vi "BIAS.vi"() -> ()   [LabVIEW 2010]
uses:
  <userlib>/bias2/subvis/Imaging_State.ctl
  <vilib>/Utility/error.llb/DialogType.ctl
  <userlib>/bias2/subvis/ROI_rect.ctl
  <userlib>/BIAS2/subvis/ExposureSettings.ctl
  <vilib>/event_ctls.llb/lveventtype.ctl
  <userlib>/BIAS2/classes/CameraBase/CameraBase.lvclass
  <vilib>/addons/h5labview/H5File.lvlib
  <vilib>/addons/h5labview/H5F_mode.ctl
  <vilib>/addons/h5labview/H5GroupObject.lvlib
  <vilib>/addons/h5labview/H5Attrib.lvlib
  <vilib>/addons/h5labview/H5Base.lvlib
  <vilib>/Analysis/NI_AALPro.lvlib
  <vilib>/Utility/file.llb/Read From Spreadsheet File (DBL).vi
  <userlib>/bias2/subvis/Frame_Controls.ctl
panel:
  in  "files":T1 caption="Files"
  in  "stop":bool
  in  "fit_buttons":cluster{"selection":bool, "stored":bool} caption="Fit"
  in  "tools_zoom":T2 caption="Zoom tools"
  in  "tools_view":cluster{"sel":bool, "in":bool, "out":bool} caption="View tools"
  in  "capture":T3 caption="Capture"
  out "stop_time":dbl=11.582550000000003
  out "busy":bool caption="Busy"
  out "recent_error":bool caption="Error"
  out "remote":bool caption="Remote"
  out "attribs":variant[](array[variant])=[variant(i32 864), variant(i32 519), variant(i32 1176), variant(i32 878), variant(i64 0), variant(string "Freerun"), variant(u32 1), variant(u32 1), variant(i64 864), variant(i64 519), variant(i64 312), variant(i64 359), variant(dbl 100000.00149011612)]
  out "acquiring":bool caption="Acquiring"
  out "img_OD":T4(plugin-control)
  out "n_atoms":dbl caption="Atom number:" format="%_4e"
  out "image_raw":sgl[][](array[numeric])
  in  "tabs":T5(tab)
  in  "newinst":bool
  in  "effective_pixel":dbl caption="effective pixel size"
  in  "rotation":u16(ring) items=["Do not rotate", "Rotate 90°", "Rotate 180°", "Rotate -90°"]
  out "cam_params":cluster{"String":string, "value":variant}[](array[cluster])=[{"String"="TriggerSource", "value"=variant(string "Freerun")}, {"String"="Timeout", "value"=variant(u32 23583)}, {"String"="ShiftPixelBits", "value"=variant(bool FALSE)}, {"String"="PixelFormat", "value"=variant(string "Mono14")}] caption="Camera Parameters"
  in  "config_cam":bool
  in  "bin_y":u8=1
  in  "bin_x":u8=1
  in  "rois":T7(array[cluster])=[{"get"=FALSE, "set"=FALSE, "rect"={"left"=0, "top"=0, "right"=0, "bottom"=0}, "color"=16777224}, {"get"=FALSE, "set"=FALSE, "rect"={"left"=0, "top"=0, "right"=0, "bottom"=0}, "color"=6618880}, {"get"=FALSE, "set"=FALSE, "rect"={"left"=0, "top"=0, "right"=0, "bottom"=0}, "color"=16776960}, {"get"=FALSE, "set"=FALSE, "rect"={"left"=0, "top"=0, "right"=0, "bottom"=0}, "color"=4849919}]
  in  "camera name":string
  out "camera model":string="GX1920 (02-2410B), serial 0xF3101FDAB"
  in  "exposure":sgl=100.0 caption="exposure (ms)"
  out "location":string caption="camera location"
  out "roi_sensor":T6={"left"=0, "top"=0, "right"=1936, "bottom"=1456} caption="camera size"
  out "keep":u8
  in  "pedestal":u16=100 caption="Camera pedestal value"
  in  "comp_Isat":bool caption="compute?"
  in  "Isat":dbl=1.5
  in  "Icutoff":dbl=500.0 caption="Intensity threshold"
  in  "xsection":dbl=2.9049e-13 caption="Transition Cross-section"
  out "working dir":path
  out "current file":string
  in  "comp_list":i32(listbox) caption="Computed Frames"
  in  "raw_ctrls":T8={"col_scheme"=0, "val_min"=100.0, "val_max"=13807.0, "automax"=TRUE} {"col_scheme" items=["Grayscale", "Rainbow", "Temperature", "-", "AlpineColors", "Amherst", "Aquamarine", "ArmyColors", "AtlanticColors", "AuroraColors", "AvocadoColors", "BeachColors", "BlueGreenYellow", "BrassTones", "BrightBands", "BrownCyanTones", "CandyColors", "CherryTones", "CMYKColors", "CoffeeTones", "DarkBands", "DarkRainbow", "DarkTerrain", "DeepSeaColors", "Default", "FallColors", "FruitPunchColors", "FuchsiaTones", "GrayTones", "GrayYellowTones", "GreenBrownTerrain", "GreenPinkTones", "IslandColors", "LabVIEW", "LakeColors", "LightTemperatureMap", "LightTerrain", "MintColors", "NeonColors", "NIST", "Pastel", "PearlColors", "PigeonTones", "PlumColors", "Rainbow", "RedBlueTones", "RedGreenSplit", "RoseColors", "RustTones", "SandyTerrain", "SiennaTones", "SolarColors", "SouthwestColors", "StarryNightColors", "SunsetColors", "TemperatureMap", "ThermometerColors", "ValentineTones", "WatermelonColors"]; "val_max" format="%_4g"; "val_min" format="%_4g"}
  in  "comp_ctrls":T8={"col_scheme"=39, "val_min"=0.0, "val_max"=3.0, "automax"=FALSE} {"col_scheme" items=["Grayscale", "Rainbow", "Temperature", "-", "AlpineColors", "Amherst", "Aquamarine", "ArmyColors", "AtlanticColors", "AuroraColors", "AvocadoColors", "BeachColors", "BlueGreenYellow", "BrassTones", "BrightBands", "BrownCyanTones", "CandyColors", "CherryTones", "CMYKColors", "CoffeeTones", "DarkBands", "DarkRainbow", "DarkTerrain", "DeepSeaColors", "Default", "FallColors", "FruitPunchColors", "FuchsiaTones", "GrayTones", "GrayYellowTones", "GreenBrownTerrain", "GreenPinkTones", "IslandColors", "LabVIEW", "LakeColors", "LightTemperatureMap", "LightTerrain", "MintColors", "NeonColors", "NIST", "Pastel", "PearlColors", "PigeonTones", "PlumColors", "Rainbow", "RedBlueTones", "RedGreenSplit", "RoseColors", "RustTones", "SandyTerrain", "SiennaTones", "SolarColors", "SouthwestColors", "StarryNightColors", "SunsetColors", "TemperatureMap", "ThermometerColors", "ValentineTones", "WatermelonColors"]; "val_max" format="%_4g"; "val_min" format="%_4g"}
  in  "raw_list":i32(listbox)=-1 caption="Raw Frames"
  in  "alpha":dbl=1.0 caption="Alpha"
  in  "hold_frames":bool caption="Hold last flat/dark frames"
  in  "histograms":bool caption="Histograms"
  in  "fit_function":enum16{"Gaussian", "ThomasFermi"}(ring)
  in  "fit clip":dbl=5.0 caption="OD clip" min=1.0
  out "fit_current":bool caption="Current"
  out "fit_number":dbl caption="Fitted atom number:"
  in  "bin_size":i32=5 caption="bin size" min=1
  out "fit_params":T9(array[cluster])=[{"param"="Fit_residuals", "uncert"=0.0, "uncert 2"=0.0}, {"param"="Fit_rebin", "uncert"=0.0, "uncert 2"=0.0}, {"param"="Gaussian_X0", "uncert"=0.12302468141779599, "uncert 2"=0.0}, {"param"="Gaussian_Y0", "uncert"=0.17648801424407168, "uncert 2"=0.0}, {"param"="Gaussian_XW", "uncert"=0.11674772619735485, "uncert 2"=0.0}, {"param"="Gaussian_YW", "uncert"=0.16283739371170114, "uncert 2"=0.0}, {"param"="Gaussian_Amp", "uncert"=0.008479207725537119, "uncert 2"=0.0}, {"param"="Gaussian_Offset", "uncert"=0.003580147540181461, "uncert 2"=0.0}, {"param"="Gaussian_Nint", "uncert"=1132011.7271960815, "uncert 2"=0.0}] caption="Fit Results" {"uncert 2" format="%#_4g"; "uncert" format="%#_4g"}
  in  "auto fit":bool caption="Auto fit"
  out "data points:":u32=7656 caption="Npoints"
  out "Y-lineout":dbl[][](graph)
  out "X-lineout":dbl[][](graph)
  in  "fit_roi":T10={"get"=FALSE, "set"=FALSE, "rect"={"left"=792, "top"=473, "right"=1233, "bottom"=911}, "color"=16711680} caption="Fitting region"
  out "recent":string[](array[string]) caption="recent log messages"
  out "state":T11 caption="system state"
  in  "last error":T12={"status"=FALSE, "code"=42, "description"="", "time"=timestamp(3029490000.67111 s since 1904-01-01)} caption="most recent error:" {"time" format="%<%H:%M:%S %d/%m/%y>T"}
  out "sequencer":T13(array[cluster])
  out "comp_data":T14(array[cluster])
  out "roi_capture":T6={"left"=686, "top"=399, "right"=1281, "bottom"=1004}
  out "roi_current":T6
  out "image_data":u16[][][](array[numeric])
  out "frame":i32=-1 caption="display_frame"
  out "fit attribs":variant[](array[variant])
  out "cam_attribs":variant
  out "BLACS port":u16
  in  "calc timeout":u32=10000
  out "raw histograms":T15(array[cluster])
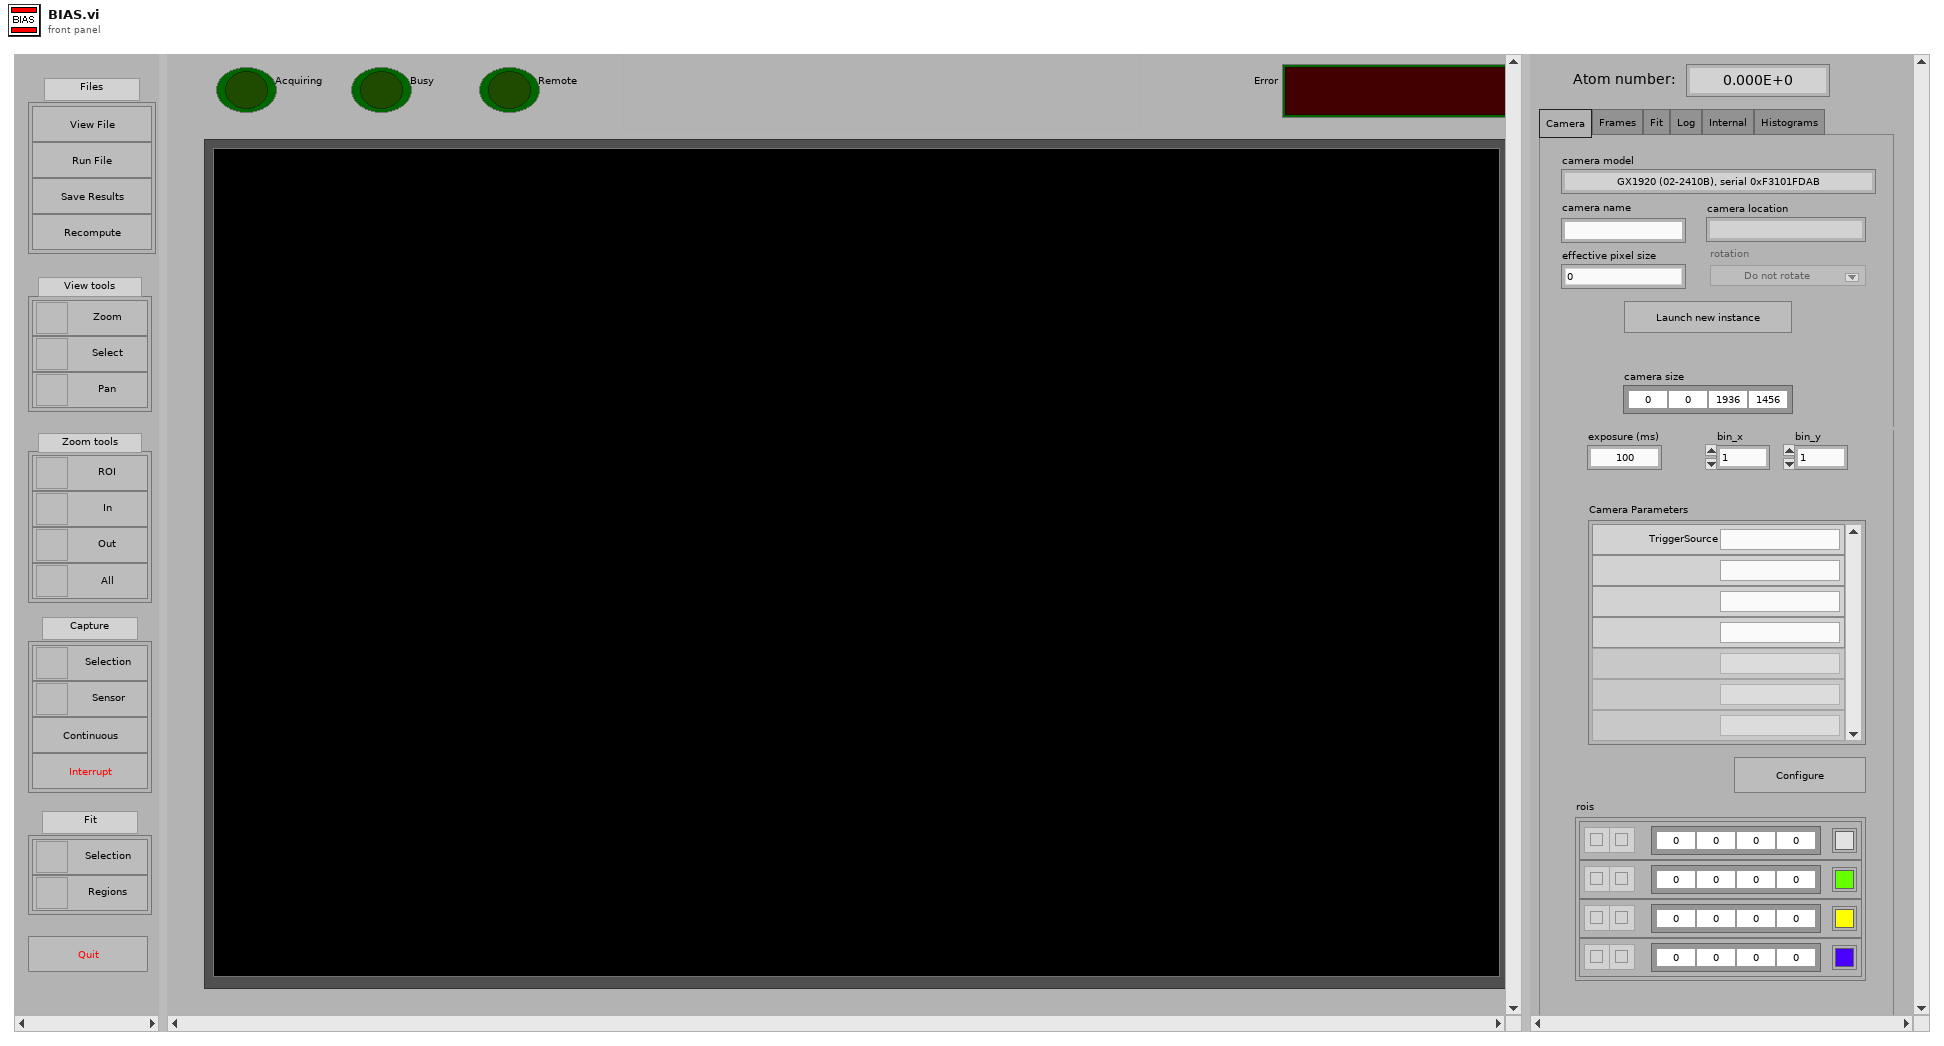
[diagram p1: front panel]
types:
  T1 = cluster{"open_file 2":bool, "open_file":bool, "save_file":bool, "open_file 3":bool}
  T2 = cluster{"sel":bool, "in":bool, "out":bool, "all":bool}
  T3 = cluster{"roi":bool, "chip":bool, "continuous":bool, "abort":bool}
  T4 = typedef "IMAQ Image.ctl" = refnum<image>
  T5 = enum32{"Camera", "Frames", "Fit", "Log", "Internal", "Histograms"}
  T6 = typedef "ROI_rect.ctl" = cluster{"left":i32, "top":i32, "right":i32, "bottom":i32}
  T7 = cluster{"get":bool, "set":bool, "rect":T6, "color":u32}[]
  T8 = typedef "Frame_Controls.ctl" = cluster{"col_scheme":u16, "val_min":sgl, "val_max":sgl, "automax":bool}
  T9 = cluster{"param":string, "uncert":dbl, "uncert 2":dbl}[]
  T10 = cluster{"get":bool, "set":bool, "rect":T6, "color":u32}
  T11 = typedef "Imaging_State.ctl" = enum16{"<NULL>", "Init", "Read File", "Save File", "Idle", "Compute", "Redraw", "Draw Overlays", "Software trigger", "Acquire", "Fit", "Clear", "Quit"}
  T12 = cluster{"status":bool, "code":i32, "description":string, "time":timestamp}
  T13 = cluster{"name":string, "shots":string[], "ids":i32[]}[]
  T14 = cluster{"sequence":string, "name":string, "data":sgl[][], "params":variant[]}[]
  T15 = cluster{"XY Graph":cluster{"X Values":dbl[], "Histogram: h(x)":i32[]}}[]
  T16 = typedef "DialogType.ctl" = u16
  T17 = typedef "zlock.ctl" = cluster{"context out":refnum<class "zmq_context.lvclass">, "endpoint":string, "timeout":u32, "name":string}
  T18 = typedef "pointer.ctl" = u64
  T19 = typedef "ExposureSettings.ctl" = cluster{"exposure":dbl, "external":bool, "roi":T6, "frames":i32, "bin_x":u8, "bin_y":u8}
  T20 = cluster{"Icutoff":dbl, "Isat":dbl, "sigma":dbl, "pixel_size":dbl}
  T21 = typedef "H5File.lvlib/H5F_mode.ctl" = enum16{"read-only", "read-write", "overwrite", "create new", "open or create"}
  T22 = enum8{"Enabled", "Disabled", "Disabled and Grayed Out"}
  T23 = typedef "Image Type" = u32
  T24 = cluster{"sensor_width":u16, "sensor_width":u16, "sensor_width":u16, "sensor_height":u16}
  T25 = cluster{"sequence":string, "name":string, "data":sgl[][], "params":variant[]}
  T26 = cluster{"X Values":dbl[], "Histogram: h(x)":i32[]}
  T27 = cluster{"Histogram Graph":cluster{"X Values":dbl[], "Histogram: h(x)":i32[]}}
  T28 = cluster{"name":string, "shots":string[], i32[]}[]
  T29 = cluster{"Name":string, "Name":string, "data":sgl[][], "params":variant[]}[]
  T30 = enum32{"Invalid", "Standard", "Closed", "Hidden", "Minimized", "Maximized"}
  T31 = typedef "lveventtype.ctl" = enum32{"Null", "Timeout", "App Instance Close", "App Instance Close?", "Autoscale Range Change", "Cell Edit", "Cell Edit?", "Cursor Grab", "Cursor Grab?", "Cursor Move", "Cursor Release", "Data Change", "Direction Change", "Display State Change", "Drag Ended", "Drag Enter", "Drag Leave", "Drag Over", "Drag Source Update", "Drag Starting", "Drag Starting?", "Drop", "Exec State Change", "Key Down", "Key Down?", "Key Repeat", "Key Repeat?", "Key Up", "Listbox Double Click", "Menu Activation?", "Menu Selection (App)", "Menu Selection? (App)", "Menu Selection (User)", "Mouse Down", "Mouse Down?", "Mouse Enter", "Mouse Leave", "Mouse Move", "Mouse Up", "NI Security User Change (App)", "Pane Size", "Panel Close", "Panel Close?", "Panel Resize", "Plot Attribute Change", "Scale Range Change", "Shortcut Menu Activation?", "Shortcut Menu Selection (App)", "Shortcut Menu Selection? (App)", "Shortcut Menu Selection (User)", "Tree Double Click", "Tree Drag", "Tree Drag?", "Tree Drop", "Tree Drop?", "Tree Item Close", "Tree Item Close?", "Tree Item Open", "Tree Item Open?", "Value Change"}
  T32 = cluster{"Global Rectangle":i32[], "Contours":cluster{"Contour Type":u32, "ROI Type":u32, "Points":i32[]}[]}
  T33 = typedef "ROI Descriptor" = cluster{"Global Rectangle":i32[], "Contours":cluster{"ID":enum32{"External", "Internal"}, "Type":u32, "Coordinates":i32[]}[]}
  T34 = cluster{"Contour Type":u32, "ROI Type":u32, "Points":i32[]}[]
  T35 = cluster{"FinalVal[0]":bool, "FinalVal[1]":bool, "FinalVal[2]":bool}
  T36 = cluster{"all rows[0]":dbl, "all rows[1]":dbl, "all rows[2]":dbl}
  T37 = cluster{"bin_x":u8, "bin_y":u8, "bin_x":u8, "bin_y":u8}
  T38 = enum16{"Standard", "Buffered", "CRLF", "Immediate"}
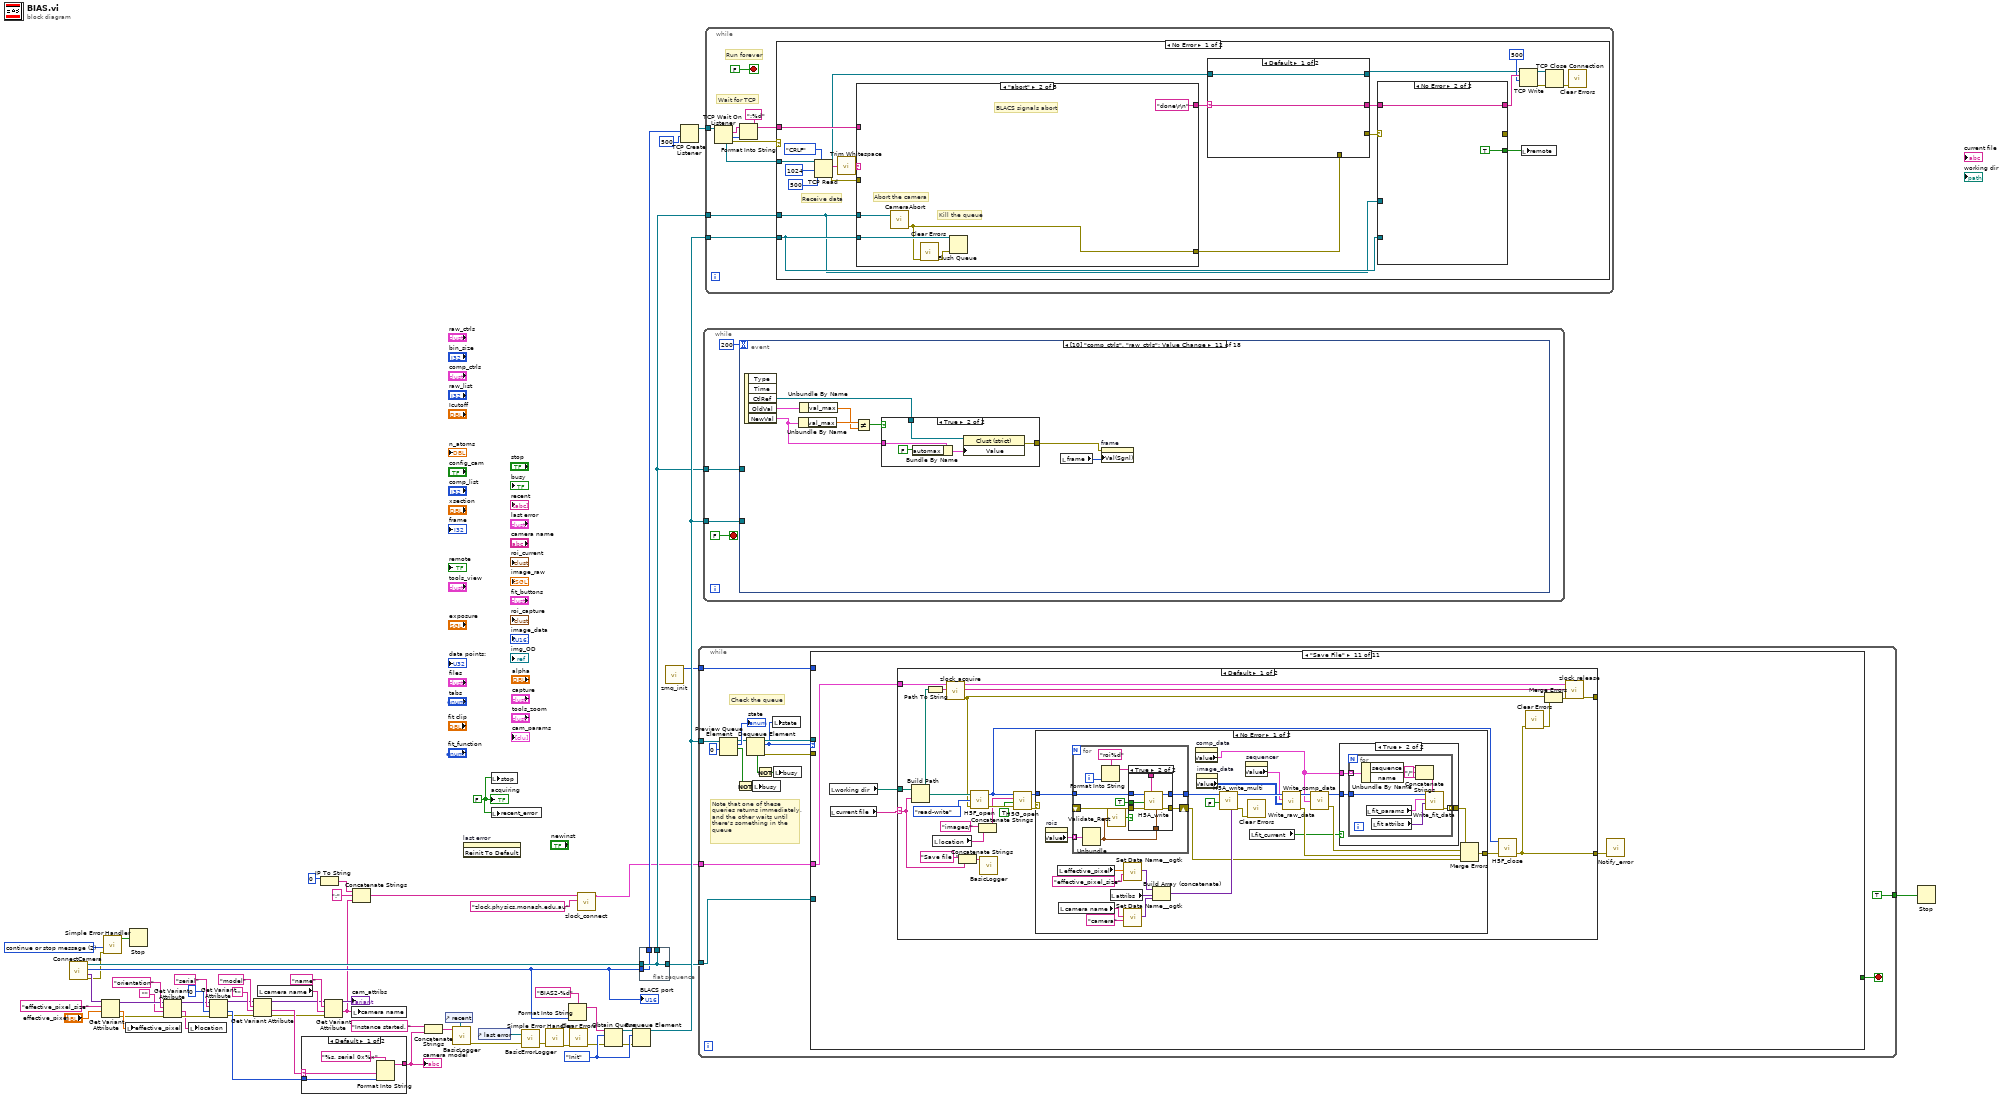
[diagram p0: block diagram]
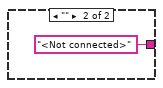
[diagram p2: hidden frame]
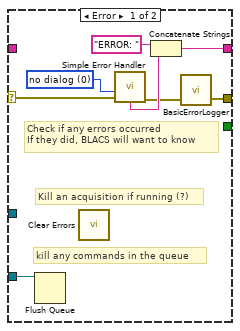
[diagram p3: hidden frame]
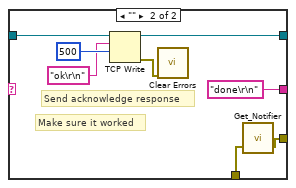
[diagram p4: hidden frame]
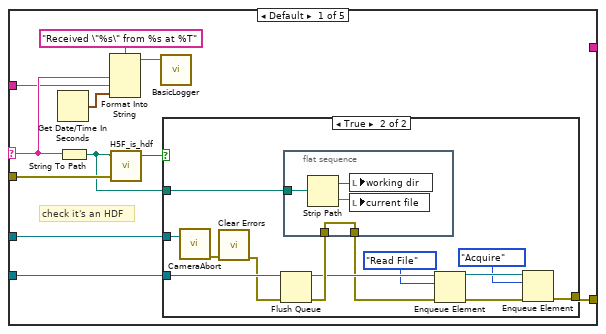
[diagram p5: hidden frame]
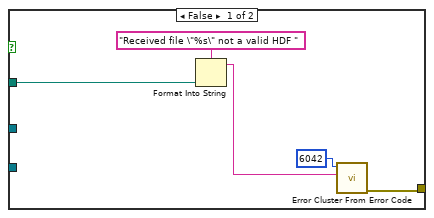
[diagram p6: hidden frame]
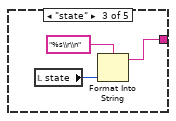
[diagram p7: hidden frame]
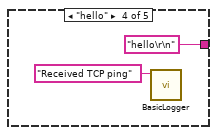
[diagram p8: hidden frame]
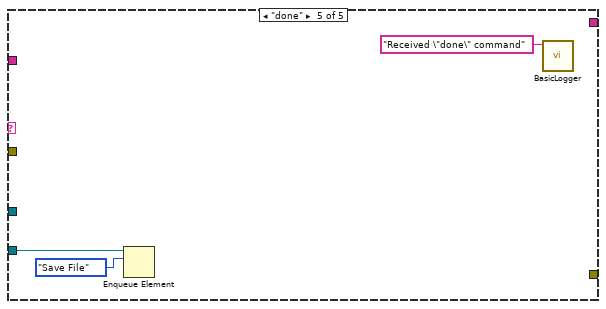
[diagram p9: hidden frame]
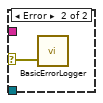
[diagram p10: hidden frame]
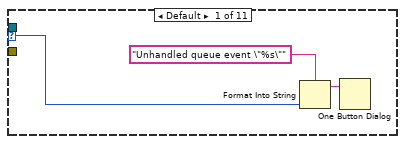
[diagram p11: hidden frame]
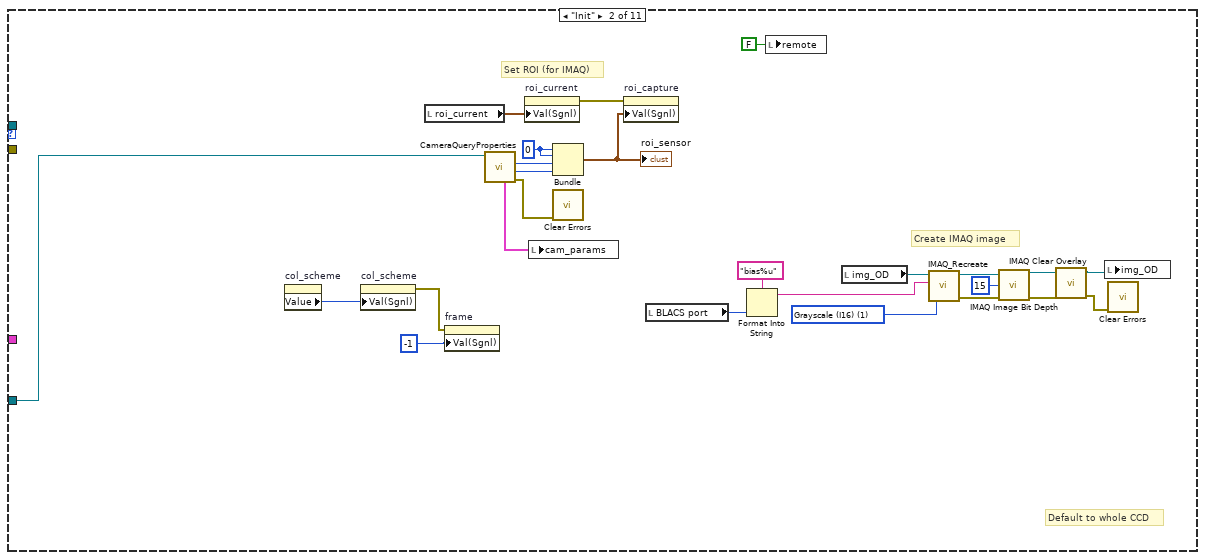
[diagram p12: hidden frame]
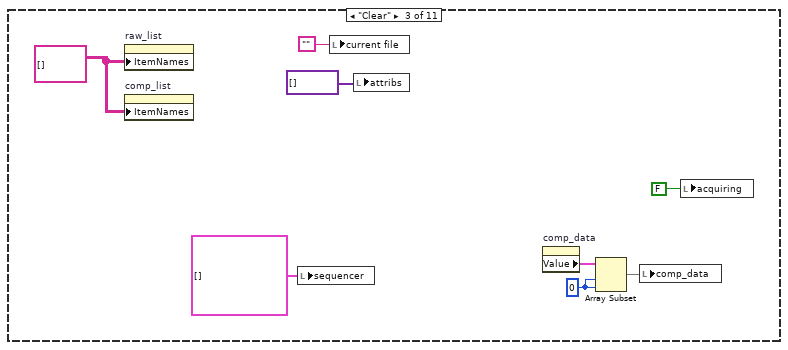
[diagram p13: hidden frame]
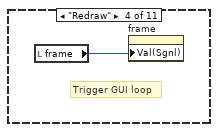
[diagram p14: hidden frame]
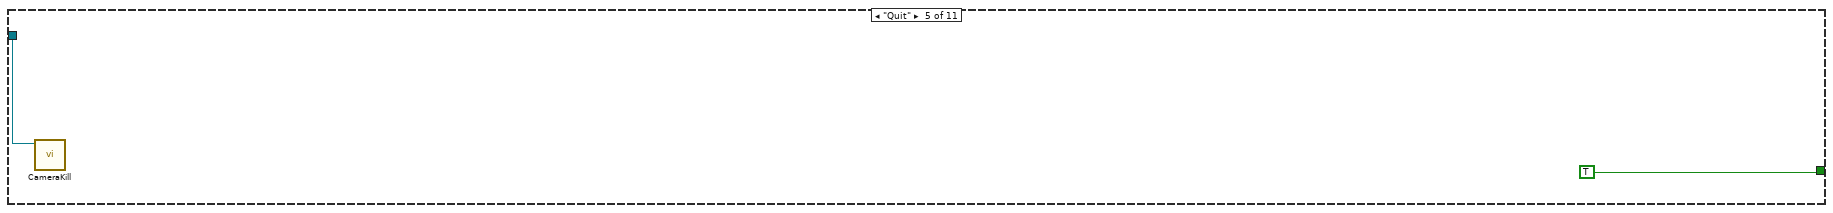
[diagram p15: hidden frame]
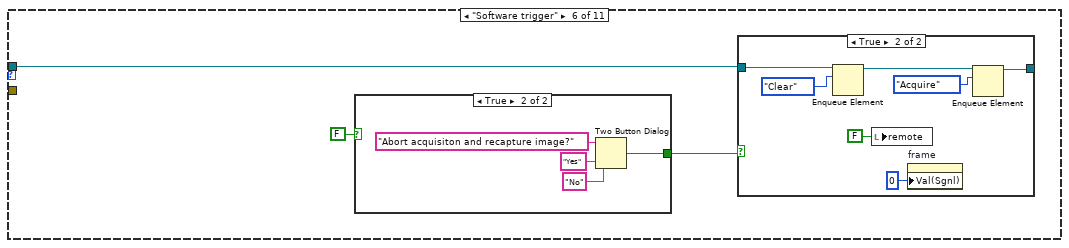
[diagram p16: hidden frame]
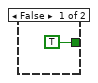
[diagram p18: hidden frame]
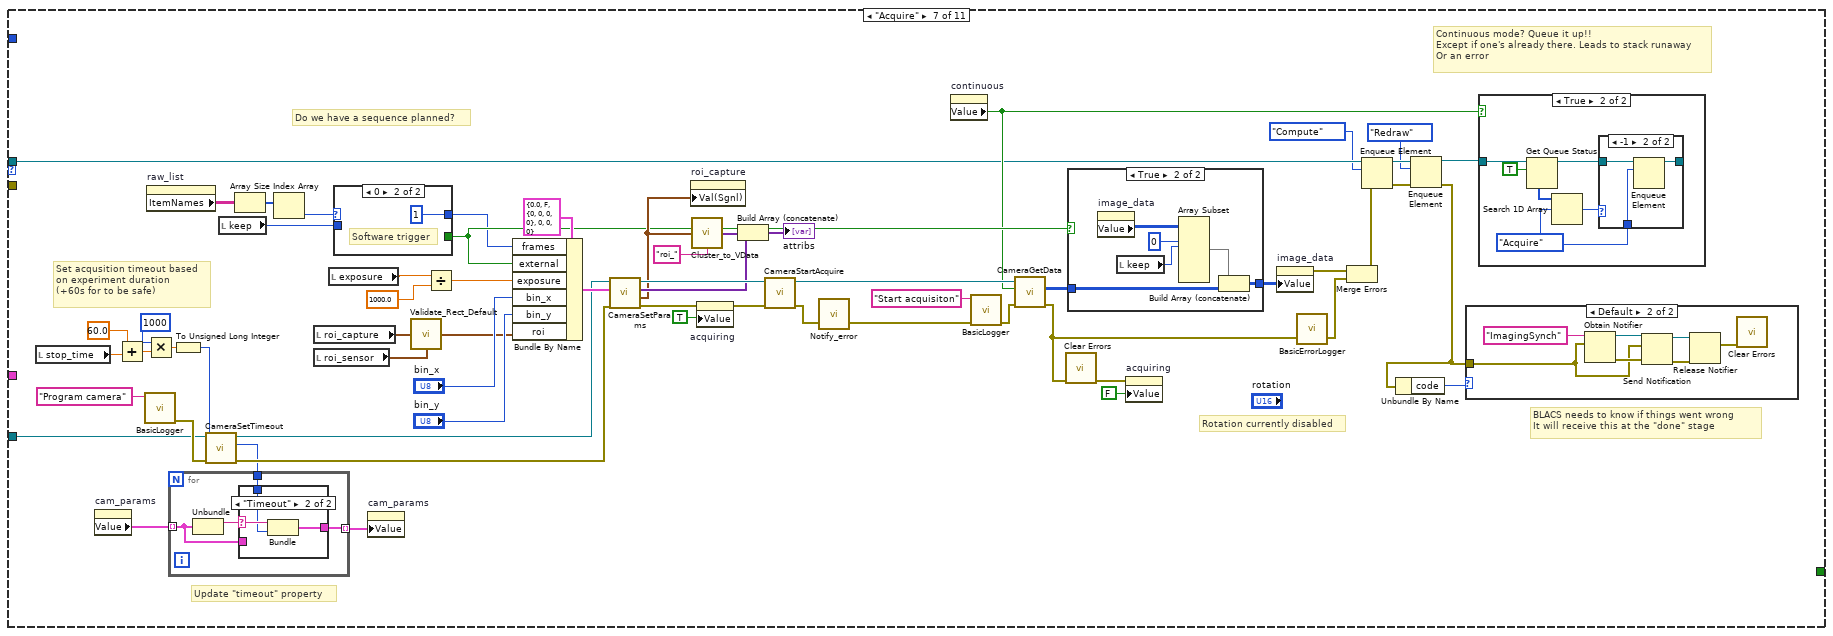
[diagram p19: hidden frame]
diagram:
  w8 = T16 2 items=["no dialog", "OK message", "continue or stop message", "OK message + warnings", "continue/stop + warnings"] ("type of dialog (OK msg:1)")
  w25 = FALSE ("acquiring")
  w58 = Imaging_State."Init" ("Imaging_State")
  n1 = call <userlib>:"ConnectCamera.vi"() -> ("error out"=w10:errorcluster, "params"=w33:variant, "port"=w20:u16, "camera"=w23:refnum<class "CameraBase.lvclass">)  [unwired: 4 in]
  "BLACS port" <- w20
  n2 = Get Variant Attribute(Variant=w33, name="effective_pixel_size", default value (empty Variant)="effective_pixel") -> (duplicate Variant=w16:variant, value=w47:dbl, error out=w13:errorcluster)  [unwired: 1 in, 1 out]
  n3 = call <vilib>:"Simple Error Handler.vi"("type of dialog (OK msg:1)"=w8, "error in (no error)"=w10) -> ("error?"=w9:bool)  [unwired: 3 in, 4 out]
  n4 = local write "effective_pixel"(w47) -> ()
  n5 = Stop(stop? (T)=w9) -> ()
  n6 = Get Variant Attribute(Variant=w16, name="orientation", default value (empty Variant)="", error in=w13) -> (duplicate Variant=w15:variant, value=w11:string, error out=w12:errorcluster)  [unwired: 1 out]
  n7 = local write "location"(w11) -> ()
  n8 = Get Variant Attribute(Variant=w15, name="serial", default value (empty Variant)=u64 0, error in=w12) -> (duplicate Variant=w30:variant, value=w32:u64, error out=w29:errorcluster)  [unwired: 1 out]
  n9 = Get Variant Attribute(Variant=w30, name="model", default value (empty Variant)="", error in=w29) -> (duplicate Variant=w28:variant, value=w31:string, error out=w27:errorcluster)  [unwired: 1 out]
  n10 = local read "camera name"() -> (w35:string)
  n11 = case shown="Default" w31 {
    selector: w31 -> [w60 _]
    tunnel: [w62 "<Not connected>"] -> w36
    tunnel: w32 -> [w61 _]
    frame Default {
      n12 = Format Into String(format string="%s, serial 0x%x", w60, w61) -> (resulting string=w62:string)  [unwired: 2 in, 1 out]
    }
    frame "" {
    }
  }
  "camera model" <- w36
  n13 = IP To String(2:u32 0 ("net address")) -> (0:w7:string)  [unwired: 1 in]
  n14 = Get Variant Attribute(Variant=w28, name="name", default value (empty Variant)=w35, error in=w27) -> (duplicate Variant=→"cam_attribs":variant, value=w4:string)  [unwired: 2 out]
  n15 = local write "camera name"(w4) -> ()
  n16 = Concatenate Strings(w7, ":" ("string"), w4) -> (w3:string)
  n17 = Concatenate Strings("Instance started, " ("string"), w36) -> (w37:string)
  n18 = control-ref of="recent"() -> (w39:refnum<vi>)
  n19 = call <userlib>:"BasicLogger.vi"("indicator"=w39, "text"=w37) -> ("error out"=w44:errorcluster)  [unwired: 5 in, 1 out]
  n20 = invoke on="last error" class="Clust (strict)" method="Reinit To Default"() -> ()  [unwired: 3 in, 3 out]
  n21 = control-ref of="last error"() -> (w52:refnum<vi>)
  n22 = local write "stop"(w25) -> ()
  n23 = local write "recent_error"(w25) -> ()
  n24 = call <userlib>:"BasicErrorLogger.vi"("error in"=w44, "indicator"=w52) -> ("error out"=w51:errorcluster)  [unwired: 1 out]
  n25 = call <vilib>:"Simple Error Handler.vi"("error in (no error)"=w51) -> ("error out"=w50:errorcluster)  [unwired: 4 in, 4 out]
  n26 = Format Into String(format string="BIAS2-%d" ("name (unnamed)"), w20) -> (resulting string=w18:string)  [unwired: 2 in, 1 out]
  n27 = call <vilib>:"Clear Errors.vi"("error in (no error)"=w50) -> ("error out"=w49:errorcluster)  [unwired: 6 in]
  n28 = call <userlib>:"zlock_connect.vi"("host"="zlock.physics.monash.edu.au", "name"=w3) -> ("zlock"=w1:T17)  [unwired: 8 in, 1 out]
  n29 = Obtain Queue(name (unnamed)=w18, element data type=w58, error in (no error)=w49) -> (queue out=w59:refnum<queue>, error out=w57:errorcluster)  [unwired: 2 in, 1 out]
  n30 = Enqueue Element(queue=w59, element=w58, error in (no error)=w57) -> (queue out=w54:refnum<queue>)  [unwired: 1 in, 2 out]
  n31 = flat-sequence {
    tunnel: w20 -> [w65]
    tunnel: w23 -> [w66]
    tunnel: [w66] -> w21
    tunnel: [w66] -> w22
    tunnel: [w65] -> w19
    frame #0 {
    }
  }
  n32 = call <vilib>:"zmq_init.vi"() -> ("context"=w34:T18)  [unwired: 4 in, 1 out]
  n33 = TCP Create Listener(9:500 ("timeout ms (25000)"), 10:w19) -> (3:w53:refnum<k5>)  [unwired: 3 in, 2 out]
  n34 = while {
    tunnel: [TRUE] -> w56
    tunnel: w22 -> [w78]
    tunnel: w54 -> [w72]
    tunnel: w34 -> [w68]
    tunnel: w1 -> [w67]
    stop <- w79 stop-if-true
    # "Check the queue"
    # "Note that one of these\nqueries returns immediately,\nand the other waits until\nthere's something in the\nqueue"
    n35 = Preview Queue Element(queue=w72, timeout in ms (-1)=0) -> (queue out=w71:refnum<queue>, element=→"state":T11, timed out?=w69:bool)  [unwired: 1 in, 1 out]
    n36 = Not(x=w69) -> (.not. x?=w70:bool)
    n37 = Dequeue Element(queue=w71) -> (queue out=w82:refnum<queue>, element=w77:T11, timed out?=w76:bool, error out=w81:errorcluster)  [unwired: 2 in]
    n38 = local write "busy"(w70) -> ()
    n39 = Not(x=w76) -> (.not. x?=w75:bool)
    n40 = local write "state"(w77) -> ()
    n41 = local write "busy"(w75) -> ()
    n42 = case shown="\"Save File\"" w77 {
      selector: w77 -> [w84 _ _ _ _ _ _ _ _ _ _]
      tunnel: w82 -> [_ _ _ _ _ w123 w145 w245 _ w414 _]
      tunnel: w81 -> [_ _ _ _ _ _ _ _ _ _ _]
      tunnel: [_ _ _ _ TRUE _ _ _ _ _ _] -> w79
      tunnel: w78 -> [_ w93 _ _ w120 _ w166 _ _ _ _]
      tunnel: w68 -> [_ _ _ _ _ _ _ w239 w330 _ _]
      tunnel: w67 -> [_ _ _ _ _ _ _ _ _ w409 w546]
      frame Default {
        n43 = Format Into String(format string="Unhandled queue event \"%s\"", w84) -> (resulting string=w83:string)  [unwired: 2 in, 1 out]
        n44 = One Button Dialog(message=w83) -> ()  [unwired: 1 in, 1 out]
      }
      frame "Init" {
        w92 = u16 0 ("sensor_width")
        w109 = T23 1 items=["Grayscale (U8)", "Grayscale (I16)", "Grayscale (SGL)", "Complex (CSG)", "RGB (U32)", "HSL (U32)", "RGB (U64)", "Grayscale (U16)"] ("type")
        # "Create IMAQ image"
        # "Default to whole CCD"
        # "Set ROI (for IMAQ)"
        n45 = property on="col_scheme" class="Ring (strict)"() -> ("Value"=w95:u16)  [unwired: 2 in, 2 out]
        n46 = property on="col_scheme" class="Ring (strict)"("Val(Sgnl)"=w95) -> (error out=w90:errorcluster)  [unwired: 2 in, 1 out]
        n47 = local read "roi_current"() -> (w104:T6)
        n48 = property on="frame" class="DigNum (strict)"(error in=w90, "Val(Sgnl)"=-1 ("display_frame")) -> ()  [unwired: 1 in, 2 out]
        n49 = call-dynamic "CameraQueryProperties.vi"("CameraBase in"=w93) -> ("error out"=w94:errorcluster, "sensor_height"=w103:u16, "sensor_width"=w102:u16, "cam_params"=w101:cluster{"String":string, "value":variant}[])  [unwired: 6 in, 1 out]
        n50 = property on="roi_current" class="Clust (strict)"("Val(Sgnl)"=w104) -> (error out=w105:errorcluster)  [unwired: 2 in, 1 out]
        n51 = local write "cam_params"(w101) -> ()
        n52 = Bundle("sensor_width"=w92, "sensor_width"=w92, "sensor_width"=w102, "sensor_height"=w103) -> (w89:T24)  [unwired: 1 in]
        "roi_sensor" <- w89
        n53 = call <vilib>:"Clear Errors.vi"("error in (no error)"=w94) -> ()  [unwired: 6 in, 1 out]
        n54 = property on="roi_capture" class="Clust (strict)"(error in=w105, "Val(Sgnl)"=w89) -> ()  [unwired: 1 in, 2 out]
        n55 = local read "BLACS port"() -> (w88:u16)
        n56 = Format Into String(format string="bias%u", w88) -> (resulting string=w86:string)  [unwired: 2 in, 1 out]
        n57 = local write "remote"(FALSE ("remote")) -> ()
        n58 = local read "img_OD"() -> (w110:T4)
        n59 = call <userlib>:"IMAQ_Recreate.vi"("type"=w109, "name"=w86, "image in"=w110) -> ("error out"=w106:errorcluster, "image out"=w108:T4)  [unwired: 3 in]
        n60 = call "IMAQ Image Bit Depth"("Image"=w108, "Bit Depth (0)"=u32 15, "error in (no error)"=w106) -> ("Image Out"=w99:T4, "error out"=w100:errorcluster)  [unwired: 10 in, 1 out]
        n61 = call "IMAQ Clear Overlay"("error in (no error)"=w100, "Image"=w99) -> ("error out"=w97:errorcluster, "Image Out"=w98:T4)  [unwired: 8 in]
        n62 = local write "img_OD"(w98) -> ()
        n63 = call <vilib>:"Clear Errors.vi"("error in (no error)"=w97) -> ()  [unwired: 6 in, 1 out]
      }
      frame "Clear" {
        w113 = 0 ("index")
        w116 = string[][] [] ("sequence")
        n64 = property on="raw_list" class="MCListbox (strict)"("ItemNames"=w116) -> ()  [unwired: 2 in, 2 out]
        n65 = property on="comp_list" class="MCListbox (strict)"("ItemNames"=w116) -> ()  [unwired: 2 in, 2 out]
        n66 = local write "sequencer"(T13 [] ("sequencer")) -> ()
        n67 = local write "current file"("") -> ()
        n68 = local write "attribs"(variant[] []) -> ()
        n69 = property on="comp_data" class="Arr (strict)"() -> ("Value"=w111:T14)  [unwired: 2 in, 2 out]
        n70 = Array Subset(array=w111, index=w113, length=w113) -> (w114:T14)
        n71 = local write "comp_data"(w114) -> ()
        n72 = local write "acquiring"(FALSE ("pending")) -> ()
      }
      frame "Redraw" {
        # "Trigger GUI loop"
        n73 = local read "frame"() -> (w119:i32)
        n74 = property on="frame" class="DigNum (strict)"("Val(Sgnl)"=w119) -> ()  [unwired: 2 in, 2 out]
      }
      frame "Quit" {
        n75 = call-dynamic "CameraKill.vi"("CameraBase in"=w120) -> ()  [unwired: 9 in, 2 out]
      }
      frame "Software trigger" {
        n76 = case shown="True" FALSE {
          tunnel: [TRUE ("T button?") w134] -> w124
          frame False {
          }
          frame True {
            n77 = Two Button Dialog(message="Abort acquisiton and recapture image?", 1:"No" ("F button name (\"Cancel\")"), 2:"Yes" ("T button name (\"OK\")")) -> (T button?=w134:bool)
          }
        }
        n78 = case shown="True" w124 {
          tunnel: [w125 w131] -> _
          tunnel: w123 -> [w125 w130]
          frame False {
          }
          frame True {
            n79 = Enqueue Element(queue=w130, element=Imaging_State."Clear") -> (queue out=w129:refnum<queue>)  [unwired: 2 in, 2 out]
            n80 = local write "remote"(FALSE ("remote")) -> ()
            n81 = property on="frame" class="DigNum (strict)"("Val(Sgnl)"=0 ("Value (Signaling)")) -> ()  [unwired: 2 in, 2 out]
            n82 = Enqueue Element(queue=w129, element=Imaging_State."Acquire") -> (queue out=w131:refnum<queue>)  [unwired: 2 in, 2 out]
          }
        }
      }
      frame "Acquire" {
        # "Update \"timeout\" property"
        # "Rotation currently disabled"
        # "Set acqusition timeout based\non experiment duration\n(+60s for to be safe)"
        # "BLACS needs to know if things went wrong\nIt will receive this at the \"done\" stage"
        # "Continuous mode? Queue it up!!\nExcept if one's already there. Leads to stack runaway\nOr an error"
        # "Do we have a sequence planned?"
        n83 = local read "stop_time"() -> (w161:dbl)
        n84 = property on="cam_params" class="Arr (strict)"() -> ("Value"=w147:cluster{"String":string, "value":variant}[])  [unwired: 2 in, 2 out]
        n85 = Add(x=60.0, y=w161) -> (x+y=w162:dbl)
        n86 = call <userlib>:"BasicLogger.vi"("text"="Program camera") -> ("error out"=w167:errorcluster)  [unwired: 6 in, 1 out]
        n87 = Multiply(x=u32 1000 ("col"), y=w162) -> (x*y=w169:dbl)
        n88 = property on="raw_list" class="MCListbox (strict)"() -> ("ItemNames"=w178:string[][])  [unwired: 2 in, 2 out]
        n89 = To Unsigned Long Integer(number=w169) -> (unsigned 32bit integer=w170:u32)
        n90 = call-dynamic "CameraSetTimeout.vi"("error in (no error)"=w167, "Timeout"=w170, "CameraBase in"=w166) -> ("error out"=w165:errorcluster, "Timeout set"=w163:u32, "CameraBase out"=w164:refnum<class "CameraBase.lvclass">)  [unwired: 6 in]
        n91 = for {
          tunnel: w147 -> [w206] mode=indexing
          tunnel: w163 -> [w207]
          tunnel: [w209] -> w146 mode=indexing
          n92 = Unbundle(w206) -> ("String"=w208:string)  [unwired: 1 out]
          n93 = case shown="\"Timeout\"" w208 {
            selector: w208 -> [_ w212]
            tunnel: [w210 w213] -> w209
            tunnel: w207 -> [_ w211]
            tunnel: w206 -> [w210 _]
            frame Default {
            }
            frame "Timeout" {
              n94 = Bundle(w212, "Timeout set"=w211) -> (w213:cluster{string, "Timeout set":u32})  [unwired: 1 in]
            }
          }
        }
        n95 = local read "keep"() -> (w171:u8)
        n96 = Array Size(array=w178) -> (size(s)=w177:i32[])
        n97 = Index Array(array=w177) -> (element=w176:i32)  [unwired: 1 in]
        n98 = local read "roi_capture"() -> (w194:T6)
        n99 = local read "roi_sensor"() -> (w189:T6)
        n100 = local read "exposure"() -> (w198:sgl)
        n101 = case shown="0" w176 {
          selector: w176 -> [w232 _]
          tunnel: [w233 1] -> w148
          tunnel: [TRUE ("external") _] -> w155
          tunnel: w171 -> [w231 _]
          frame Default {
            n102 = Subtract(x=w232, y=w231) -> (x-y=w233:i32)
          }
          frame 0 {
            # "Software trigger"
          }
        }
        n103 = property on="cam_params" class="Arr (strict)"("Value"=w146) -> ()  [unwired: 2 in, 2 out]
        n104 = call <userlib>:"Validate_Rect_Default.vi"("rect"=w194, "default"=w189) -> ("out"=w152:T6)
        n105 = Divide(x=w198, y=sgl 1000.0) -> (x/y=w193:sgl)
        n106 = Bundle By Name(cluster=T19 {"exposure"=0.0, "external"=FALSE, "roi"={"left"=0, "top"=0, "right"=0, "bottom"=0}, "frames"=0, "bin_x"=0, "bin_y"=0} ("settings"), "frames"=w148, "external"=w155, "exposure"=w193, "bin_x"="bin_x", "bin_y"="bin_y", "roi"=w152) -> (w192:T19)
        n107 = call-dynamic "CameraSetParams.vi"("error in (no error)"=w165, "settings"=w192, "CameraBase in"=w164) -> ("error out"=w183:errorcluster, "roi_out"=w157:T6, "attributes"=w175:variant[], "CameraBase out"=w182:refnum<class "CameraBase.lvclass">)  [unwired: 5 in]
        n108 = property on="roi_capture" class="Clust (strict)"("Val(Sgnl)"=w157) -> ()  [unwired: 2 in, 2 out]
        n109 = call <userlib>:"Cluster_to_VData.vi"("cluster"=w157, "prefix"="roi_") -> ("vdata"=w174:variant[])
        n110 = property on="acquiring" class="Bool (strict)"(error in=w183, "Value"=TRUE ("acquiring")) -> (error out=w180:errorcluster)  [unwired: 1 in, 1 out]
        n111 = Build Array (concatenate)(w174, w175) -> (→"attribs":variant[])
        n112 = call-dynamic "CameraStartAcquire.vi"("error in (no error)"=w180, "CameraBase in"=w182) -> ("error out"=w159:errorcluster, "CameraBase out"=w181:refnum<class "CameraBase.lvclass">)  [unwired: 8 in]
        n113 = call <userlib>:"Notify_error.vi"("error in"=w159) -> ("error out"=w154:errorcluster)  [unwired: 2 in]
        n114 = property on="continuous" class="Bool (strict)"() -> ("Value"=w151:bool)  [unwired: 2 in, 2 out]
        n115 = call <userlib>:"BasicLogger.vi"("error in"=w154, "text"="Start acquisiton") -> ("error out"=w179:errorcluster)  [unwired: 5 in, 1 out]
        n116 = call-dynamic "CameraGetData.vi"("error in (no error)"=w179, "keep open?"=w151, "CameraBase in"=w181) -> ("error out"=w196:errorcluster, "image_data"=w156:u16[][][])  [unwired: 6 in, 1 out]
        n117 = call <vilib>:"Clear Errors.vi"("error in (no error)"=w196) -> ("error out"=w186:errorcluster)  [unwired: 6 in]
        n118 = case shown="True" w155 {
          tunnel: [w199 w202] -> w158
          tunnel: w156 -> [w199 w200]
          frame False {
          }
          frame True {
            n119 = property on="image_data" class="Arr (strict)"() -> ("Value"=w201:u16[][][])  [unwired: 2 in, 2 out]
            n120 = local read "keep"() -> (w204:u8)
            n121 = Array Subset(array=w201, index (dim 0)=0 ("index"), length (dim 0)=w204) -> (w203:u16[][][])  [unwired: 4 in]
            n122 = Build Array (concatenate)(w203, w200) -> (w202:u16[][][])
          }
        }
        n123 = property on="acquiring" class="Bool (strict)"(error in=w186, "Value"=FALSE ("acquiring")) -> ()  [unwired: 1 in, 2 out]
        n124 = property on="image_data" class="Arr (strict)"("Value"=w158) -> (error out=w150:errorcluster)  [unwired: 2 in, 1 out]
        n125 = call <userlib>:"BasicErrorLogger.vi"("error in"=w196) -> ("error out"=w149:errorcluster)  [unwired: 1 in, 1 out]
        n126 = Merge Errors(w150, w149) -> (w140:errorcluster)
        n127 = Enqueue Element(queue=w145, element=Imaging_State."Compute", error in (no error)=w140) -> (queue out=w143:refnum<queue>, error out=w139:errorcluster)  [unwired: 1 in, 1 out]
        n128 = Enqueue Element(queue=w143, element=Imaging_State."Redraw", error in (no error)=w139) -> (queue out=w144:refnum<queue>, error out=w138:errorcluster)  [unwired: 1 in, 1 out]
        n129 = Unbundle By Name(w138) -> ("code"=w172:i32)
        n130 = case shown="Default" w172 {
          tunnel: w138 -> [_ w214]
          frame 0, 5024 {
            # "Fine or Abort"
          }
          frame Default {
            n131 = Obtain Notifier(name (unnamed)="ImagingSynch", notification data type=w214) -> (notifier out=w217:refnum<notifier>, error out=w218:errorcluster)  [unwired: 2 in, 1 out]
            n132 = Send Notification(notification=w214, notifier=w217, error in (no error)=w218) -> (notifier out=w220:refnum<notifier>, error out=w219:errorcluster)
            n133 = Release Notifier(notifier=w220, error in (no error)=w219) -> (last notification=w215:errorcluster)  [unwired: 1 in, 2 out]
            n134 = call <vilib>:"Clear Errors.vi"("error in (no error)"=w215) -> ()  [unwired: 6 in, 1 out]
          }
        }
        n135 = case shown="True" w151 {
          tunnel: w144 -> [_ w226]
          frame False {
          }
          frame True {
            w221 = Imaging_State."Acquire" ("element")
            n136 = Get Queue Status(queue=w226, return elements? (F)=TRUE) -> (queue out=w222:refnum<queue>, elements=w224:T11[])  [unwired: 1 in, 6 out]
            n137 = Search 1D Array(1D array=w224, element=w221) -> (index of element=w223:i32)  [unwired: 1 in]
            n138 = case shown="-1" w223 {
              tunnel: [w227 w230] -> _
              tunnel: w222 -> [w227 w229]
              tunnel: w221 -> [_ w228]
              frame Default {
              }
              frame -1 {
                n139 = Enqueue Element(queue=w229, element=w228) -> (queue out=w230:refnum<queue>)  [unwired: 2 in, 2 out]
              }
            }
          }
        }
      }
      frame "Compute" {
        # ">> num frames >>"
        # "Ensure the fit happens before saving if auto fit enabled."
        n140 = property on="comp_data" class="Arr (strict)" props=["Value"]() -> ()  [unwired: 2 in, 3 out]
        n141 = property on="sequencer" class="Arr (strict)"() -> ("Value"=w240:T13)  [unwired: 2 in, 2 out]
        n142 = property on="raw_list" class="MCListbox (strict)"() -> ("ItemNames"=w248:string[][])  [unwired: 2 in, 2 out]
        n143 = for {
          N -> [w274]
          tunnel: w240 -> [w278] mode=indexing
          tunnel: [w284] -> w243
          tunnel: w248 -> [w281]
          tunnel: [errorcluster {"status"=FALSE, "code"=0, "source"=""} ("error in (no error)")] -> w244
          tunnel: [w274] -> w246
          tunnel: w239 -> [w273]
          shift-right: [w271] -> w237
          shift-left: T14 [] -> [w272]
          # ">> sequence >>"
          # "Try to find frames"
          n144 = Unbundle(w278) -> ("name"=w285:string)  [unwired: 2 out]
          n145 = call <userlib>:"Keep_Find.vi"("x"="atoms" ("name"), "sequence"=w278) -> ("index"=w276:i32)  [unwired: 1 in]
          n146 = call <userlib>:"Keep_Find.vi"("x"="flat" ("name"), "rawlist"=w281, "sequence"=w278) -> ("index"=w280:i32)
          n147 = call <userlib>:"Keep_Find.vi"("x"="dark" ("name"), "rawlist"=w281, "sequence"=w278) -> ("index"=w279:i32)
          n148 = Greater Or Equal To 0?(x=w276) -> (x >= 0?=w288:bool)
          n149 = Greater Or Equal To 0?(x=w280) -> (x >= 0?=w287:bool)
          n150 = Compound Arithmetic op=AND(w288, w287) -> (w286:bool)
          n151 = case shown="True" w286 {
            tunnel: w276 -> [_ w326]
            tunnel: w280 -> [_ w324]
            tunnel: w279 -> [_ w325]
            tunnel: w285 -> [_ w323]
            tunnel: [_ w313] -> w284
            tunnel: w273 -> [_ w295]
            tunnel: w272 -> [w289 w290]
            tunnel: [w289 w291] -> w271
            frame False {
            }
            frame True {
              w302 = 1 ("dimension size")
              n152 = property on="image_data" class="Arr (strict)"() -> ("Value"=w306:u16[][][])  [unwired: 2 in, 2 out]
              n153 = local read "effective_pixel"() -> (w293:dbl)
              n154 = Index Array(array=w306, index (dim 0) #1=w326, index (dim 0) #2=w324, index (dim 0) #3=w325) -> (element #1=w296:u16[][], element #2=w297:u16[][], element #3=w299:u16[][])  [unwired: 6 in]
              n155 = local read "xsection"() -> (w310:dbl)
              n156 = Select(t="Isat", s="comp_Isat", f=0.0) -> (s? t:f=w311:dbl)
              n157 = local read "Icutoff"() -> (w312:dbl)
              n158 = Empty Array?(array=w299) -> (empty?=w301:bool)
              n159 = Initialize Array("pedestal", w302, w302) -> (w300:u16[][])
              n160 = Bundle By Name(cluster=T20 {"Icutoff"=0.0, "Isat"=0.0, "sigma"=0.0, "pixel_size"=0.0} ("params"), "Icutoff"=w312, "Isat"=w311, "sigma"=w310, "pixel_size"=w293) -> (w304:T20)
              n161 = Select(t=w300, s=w301, f=w299) -> (s? t:f=w298:u16[][])
              n162 = call <userlib>:"Compute_OD.vi"("timeout"="calc timeout", "params"=w304, "dark"=w298, "flat"=w297, "atoms"=w296, "ctx in"=w295) -> ("error out"=w309:errorcluster, "alpha"=w315:dbl, "N"=w313:dbl, "OD"=w314:sgl[][])
              n163 = call <userlib>:"BasicErrorLogger.vi"("error in"=w309) -> ("error out"=w321:errorcluster)  [unwired: 1 in, 1 out]
              n164 = call <vilib>:"Clear Errors.vi"("error in (no error)"=w321) -> ()  [unwired: 6 in, 1 out]
              n165 = local write "alpha"(w315) -> ()
              n166 = call <userlib>:"Set Data Name__ogtk.vi"("Data Name"="atom_number", "Data"=w313) -> ("Renamed Data"=w317:variant)  [unwired: 8 in, 1 out]
              n167 = property class="Clust (strict)"() -> ("Value"=w320:T25)  [unwired: 2 in, 2 out]
              n168 = Build Array(w317) -> (w318:variant[])
              n169 = Bundle(cluster=w320, "sequence"=w323, "name"="OD", "data"=w314, "params"=w318) -> (w292:T25)
              n170 = Build Array (concatenate)(w290, w292) -> (w291:T14)
            }
          }
        }
        "comp_data" <- w237
        n171 = case shown="Default" w246 {
          tunnel: w244 -> [_ w251]
          frame Default {
            n172 = local read "frame"() -> (w250:i32)
            n173 = property on="frame" class="DigNum (strict)"("Val(Sgnl)"=w250) -> ()  [unwired: 2 in, 2 out]
          }
          frame 1.. {
            n174 = property on="comp_list" class="MCListbox (strict)"(error in=w251, "Val(Sgnl)"=0 ("Value (Signaling)")) -> ()  [unwired: 1 in, 2 out]
          }
        }
        n175 = Greater Than 0?(x=w243) -> (x > 0?=w241:bool)
        n176 = for {
          tunnel: w237 -> [w270] mode=indexing
          tunnel: [w269] -> w249 mode=indexing
          n177 = Unbundle(w270) -> ("sequence"=w268:string, "name"=w267:string)  [unwired: 2 out]
          n178 = Build Array(w268, w267) -> (w269:string[])
        }
        n179 = call <userlib>:"GrayOut.vi"("enabled?"=w241) -> ("state"=w242:T22)
        n180 = case shown="True" "histograms" {
          frame False {
          }
          frame True {
            # "Raw image histograms (very slow)"
            n181 = property on="image_data" class="Arr (strict)"() -> ("Value"=w253:u16[][][])  [unwired: 2 in, 2 out]
            n182 = for {
              tunnel: w253 -> [w261] mode=indexing
              tunnel: [w257] -> w254 mode=indexing
              n183 = Array Size(array=w261) -> (size(s)=w263:i32[])
              n184 = Multiply Array Elements(1:w263) -> (0:w262:i32)
              n185 = Reshape Array(w261, w262) -> (w260:u16[])
              n186 = call <vilib>:"General Histogram.vi"("X"=w260, "max"=16384.0, "min"=0.0, "# bins"=400 ("intervals")) -> ("Histogram Graph"=w258:T26)  [unwired: 7 in, 4 out]
              n187 = Bundle("Histogram Graph"=w258) -> (w257:T27)  [unwired: 1 in]
            }
            "raw histograms" <- w254
          }
        }
        n188 = property on="n_atoms" class="DigNum (strict)"("Value"=w243, "DisabledEnum"=w242) -> ()  [unwired: 2 in, 2 out]
        n189 = case shown="True" "auto fit" {
          tunnel: w245 -> [_ w266]
          tunnel: w244 -> [_ w264]
          frame False {
          }
          frame True {
            n190 = Enqueue Element At Opposite End(queue=w266, element=Imaging_State."Fit", error in (no error)=w264) -> ()  [unwired: 1 in, 3 out]
          }
        }
        n191 = property on="comp_list" class="MCListbox (strict)"("ItemNames"=w249) -> ()  [unwired: 2 in, 2 out]
      }
      frame "Fit" {
        n192 = property on="comp_data" class="Arr (strict)"() -> ("Value"=w332:T14)  [unwired: 2 in, 2 out]
        n193 = local read "frame"() -> (w343:i32)
        n194 = property on="image_data" class="Arr (strict)"() -> ("Value"=w333:u16[][][])  [unwired: 2 in, 2 out]
        n195 = local read "fit_roi"() -> (w354:T10)
        n196 = local read "roi_capture"() -> (w350:T6)
        n197 = Unbundle By Name(w354) -> ("rect"=w336:T6)
        n198 = Max & Min(x=w343, y=0) -> (max(x,y)=w341:i32)  [unwired: 1 out]
        n199 = Empty Array?(array=w332) -> (empty?=w347:bool)
        n200 = call <userlib>:"Validate_Rect_Default.vi"("rect"=w336, "default"=w350) -> ("out"=w334:T6)
        n201 = Index Array(array=w332) -> (element=w352:T25)  [unwired: 1 in]
        n202 = Index Array(array=w333, index (dim 0)=w341) -> (element=w344:u16[][])  [unwired: 2 in]
        n203 = Negate(x=w350) -> (-x=w349:T6)
        n204 = Unbundle By Name(w352) -> ("data"=w346:sgl[][])
        n205 = call <userlib>:"Apply_Rect_Offset.vi"("offset rect"=w349, "input"=w334) -> ("output"=w335:T6)  [unwired: 3 in]
        n206 = Select(t=w344, s=w347, f=w346) -> (s? t:f=w345:sgl[][])
        n207 = Unbundle(w335) -> ("left"=w338:i32, "top"=w337:i32, "right"=w360:i32, "bottom"=w359:i32)
        n208 = Subtract(x=w359, y=w337) -> (x-y=w358:i32)
        n209 = Subtract(x=w360, y=w338) -> (x-y=w357:i32)
        n210 = local read "fit_function"() -> (w328:enum16{"Gaussian", "ThomasFermi"})
        n211 = Array Subset(array=w345, index (row)=w337, length (row)=w358, index (col)=w338, length (col)=w357) -> (w356:sgl[][])
        n212 = Array Size(array=w356) -> (size(s)=w355:i32[])
        n213 = Format Into String(w328) -> (resulting string=w327:string)  [unwired: 3 in, 1 out]
        n214 = Multiply Array Elements(1:w355) -> (0:w329:i32)
        n215 = call <vilib>:"Set Busy.vi"("disable click? (T)"=FALSE) -> ("error out"=w348:errorcluster)  [unwired: 9 in, 1 out]
        n216 = Greater Than 0?(x=w329) -> (x > 0?=w353:bool)
        n217 = case shown="True" w353 {
          tunnel: w356 -> [_ w381]
          tunnel: w335 -> [_ w389]
          tunnel: w348 -> [_ _]
          tunnel: [_ TRUE] -> w340
          tunnel: [errorcluster {"status"=FALSE, "code"=0, "source"=""} ("error in (no error)") _] -> w331
          tunnel: w330 -> [_ w376]
          tunnel: w329 -> [_ w373]
          tunnel: w327 -> [_ w366]
          frame False {
          }
          frame True {
            n218 = Square Root(x=w373) -> (sqrt(x)=w372:dbl)
            n219 = Divide(x=w372, y=200 ("fit_rebin")) -> (x/y=w370:dbl)
            n220 = Round To Nearest(number=w370) -> (nearest integer value=w364:dbl)
            n221 = local read "fit clip"() -> (w368:dbl)
            n222 = local read "calc timeout"() -> (w369:u32)
            n223 = Max & Min(x=w364, y=1.0) -> (max(x,y)=w362:dbl)  [unwired: 1 out]
            n224 = call <userlib>:"Compute_Fit.vi"("timeout"=w369, "clip"=w368, "binsize"=w362, "fit_function"=w366, "data"=w381, "ctx in"=w376) -> ("error out"=w396:errorcluster, "Y_section"=→"Y-lineout":dbl[][], "X_section"=→"X-lineout":dbl[][], "fit"=w382:variant)  [unwired: 1 in]
            n225 = local write "bin_size"(w362) -> ()
            n226 = Get Variant Attribute(Variant=w382) -> (duplicate Variant=w380:variant, names=w395:string[])  [unwired: 3 in, 2 out]
            n227 = for {
              tunnel: [w408] -> w393 mode=indexing
              tunnel: w395 -> [w402] mode=indexing
              tunnel: w380 -> [w407]
              tunnel: dbl[] [] -> [w406]
              n228 = Get Variant Attribute(Variant=w407, name=w402, default value (empty Variant)=w406) -> (value=w405:dbl[])  [unwired: 1 in, 3 out]
              n229 = Index Array(array=w405) -> (element #1=w404:dbl, element #2=w403:dbl)  [unwired: 2 in]
              n230 = Bundle(w402, w404, w403) -> (w408:cluster{string, dbl, dbl})  [unwired: 1 in]
            }
            "fit_params" <- w393
            n231 = call <userlib>:"BasicErrorLogger.vi"("error in"=w396) -> ("error out"=w401:errorcluster)  [unwired: 1 in, 1 out]
            n232 = Unbundle By Name(w389) -> ("left"=w390:i32, "top"=w386:i32)
            n233 = call <vilib>:"Clear Errors.vi"("error in (no error)"=w401) -> ()  [unwired: 6 in, 1 out]
            n234 = call <userlib>:"Set Data Name__ogtk.vi"("Data Name"="fit_offset_X", "Data"=w390) -> ("Renamed Data"=w385:variant)  [unwired: 8 in, 1 out]
            n235 = call <userlib>:"Set Data Name__ogtk.vi"("Data Name"="fit_offset_Y", "Data"=w386) -> ("Renamed Data"=w384:variant)  [unwired: 8 in, 1 out]
            n236 = local read "effective_pixel"() -> (w400:dbl)
            n237 = local read "xsection"() -> (w397:dbl)
            n238 = Build Array(w385, w384) -> (→"fit attribs":variant[])
            n239 = Concatenate Strings(w366, "_Nint" ("Data Name")) -> (w365:string)
            n240 = Square(x=w400) -> (x^2=w399:dbl)
            n241 = Get Variant Attribute(Variant=w380, name=w365, default value (empty Variant)=dbl[] []) -> (value=w379:dbl[], error out=w377:errorcluster)  [unwired: 1 in, 2 out]
            n242 = Index Array(array=w379) -> (element=w375:dbl)  [unwired: 1 in]
            n243 = Compound Arithmetic op=MULTIPLY(w375, w399, invert w397) -> (→"fit_number":dbl)
            n244 = call <vilib>:"Clear Errors.vi"("error in (no error)"=w377) -> ()  [unwired: 6 in, 1 out]
          }
        }
        "fit_current" <- w340
        n245 = call <vilib>:"Unset Busy.vi"("error in (no error)"=w331) -> ()  [unwired: 10 in, 1 out]
        n246 = property on="fit_buttons" class="Clust (strict)"("Value"=cluster{"selection":bool, "stored":bool} {"selection"=FALSE, "stored"=FALSE} ("fit_buttons")) -> ()  [unwired: 2 in, 2 out]
      }
      frame "Read File" {
        n247 = local write "recent_error"(FALSE ("recent_error")) -> ()
        n248 = local read "working dir"() -> (w413:path)
        n249 = local read "current file"() -> (w412:string)
        n250 = property on="continuous" class="Bool (strict)"("Value"=FALSE ("continuous")) -> ()  [unwired: 2 in, 2 out]
        n251 = case shown="Default" w412 {
          selector: w412 -> [w445 _]
          tunnel: w414 -> [w451 _]
          tunnel: w413 -> [w446 _]
          tunnel: w409 -> [w422 _]
          tunnel: [w415 _] -> _
          frame Default {
            n252 = local read "camera name"() -> (w448:string)
            n253 = Build Path(base path=w446, name or relative path=w445) -> (appended path=w423:path)
            n254 = Path To String(path=w423) -> (string=w424:string)
            n255 = call <userlib>:"zlock_acquire.vi"("key"=w424, "ZLock in"=w422) -> ("error out"=w416:errorcluster, "key out"=w420:string, "ZLock out"=w421:T17)  [unwired: 7 in]
            n256 = Concatenate Strings("Read file  " ("text"), w445) -> (w450:string)
            n257 = call <vilib>:"H5F_open.vi"("error in (no error)"=w416, "mode"=H5F_mode."read-only", "path"=w423) -> ("error out"=w433:errorcluster, "ref"=w430:i32)  [unwired: 1 in]
            n258 = Concatenate Strings("/devices/" ("Name"), w448) -> (w429:string)
            n259 = call <userlib>:"BasicLogger.vi"("text"=w450) -> ()  [unwired: 6 in, 2 out]
            n260 = call <vilib>:"H5G_open.vi"("error in (no error)"=w433, "name"=w429, "ref"=w430) -> ("error out"=w432:errorcluster, "group"=w431:i32)  [unwired: 3 in]
            n261 = case shown="No Error" w432 {
              selector: w432 -> [_ w534]
              tunnel: [w506 w533] -> w439
              tunnel: w431 -> [w483 _]
              tunnel: [w503 w536] -> w440
              tunnel: [w505 w531] -> w435
              tunnel: [w492 w532] -> w438
              tunnel: [w499 w537] -> w437
              tunnel: w430 -> [w496 w536]
              frame No Error {
                w511 = "EXPOSURES" ("name")
                # "When is the experiment scheduled to finish? (for setting timeout)"
                n262 = call <vilib>:"H5A_read_dbl.vi"("attrib_name"="exposure_time" ("attribute"), "ref"=w483) -> ("error out"=w480:errorcluster, "ref out"=w482:i32, "value"=w478:dbl)  [unwired: 5 in]
                n263 = Multiply(x=w478, y=1000.0) -> (x*y=w507:dbl)
                n264 = local write "exposure"(w507) -> ()
                n265 = call <vilib>:"H5A_read_str.vi"("attrib_name"="orientation" ("attribute"), "error in (no error)"=w480, "ref"=w482) -> ("error out"=w476:errorcluster, "ref out"=w509:i32, "value"=w477:string)  [unwired: 4 in]
                "location" <- w477
                n266 = Concatenate Strings("/images/" ("Name"), w477) -> (w497:string)
                n267 = call <vilib>:"H5D_read_col_str.vi"("column"=u16 2, "error in (no error)"=w476, "table"=w511, "ref"=w509) -> ("error out"=w489:errorcluster, "ref out"=w512:i32, "data"=w488:string[])  [unwired: 2 in, 1 out]
                n268 = call <vilib>:"H5D_read_col_str.vi"("column"=u16 0, "error in (no error)"=w489, "table"=w511, "ref"=w512) -> ("error out"=w490:errorcluster, "ref out"=w508:i32, "data"=w486:string[])  [unwired: 2 in, 1 out]
                n269 = call <vilib>:"H5G_close.vi"("error in (no error)"=w490, "ref"=w508) -> ("error out"=w502:errorcluster)  [unwired: 3 in]
                n270 = property on="image_data" class="Arr (strict)"() -> ("Value"=w485:u16[][][])  [unwired: 2 in, 2 out]
                n271 = property on="raw_list" class="MCListbox (strict)"() -> ("ItemNames"=w501:string[][])  [unwired: 2 in, 2 out]
                n272 = call <vilib>:"H5L_exists.vi"("path"=w497, "loc_id"=w496) -> ("path out"=w491:string, "exists?"=w498:bool, "loc_id out"=w495:i32)  [unwired: 1 in, 1 out]
                n273 = call <userlib>:"Fix Sequence.vi"("sequences"=w486, "shots"=w488, "old sequence list"=w501, "image_data"=w485, "keep?"="hold_frames") -> ("sequencer"=w499:T28, "held data"=w494:u16[][][])
                n274 = case shown="True" w498 {
                  tunnel: [w515 w529] -> w506
                  tunnel: w491 -> [_ w528]
                  tunnel: [_ w527] -> w505
                  tunnel: [_ w526] -> w493
                  tunnel: w495 -> [_ w518]
                  tunnel: w502 -> [w515 w517]
                  tunnel: w499 -> [_ w516]
                  frame False {
                  }
                  frame True {
                    n275 = call <vilib>:"H5G_open.vi"("error in (no error)"=w517, "name"=w528, "ref"=w518) -> ("error out"=w524:errorcluster, "group"=w525:i32)  [unwired: 3 in]
                    n276 = local read "roi_capture"() -> (w520:T6)
                    n277 = call <userlib>:"Read_Exposures.vi"("ref in"=w525, "sequencer"=w516, "error in"=w524) -> ("ref out"=w522:i32, "ROI"=w521:T6, "loaded images"=w526:u16[][][], "computations"=w527:T29, "error out"=w523:errorcluster)  [unwired: 1 in]
                    n278 = call <userlib>:"Validate_Rect_Default.vi"("rect"=w521, "default"=w520) -> ("out"=w519:T6)
                    n279 = local write "roi_capture"(w519) -> ()
                    n280 = call <vilib>:"H5G_close.vi"("error in (no error)"=w523, "ref"=w522) -> ("error out"=w529:errorcluster)  [unwired: 3 in]
                  }
                }
                n281 = call <vilib>:"H5A_read_dbl.vi"("attrib_name"="stop_time" ("attribute"), "obj_name"="/devices/pulseblaster_0" ("Name"), "ref"=w496) -> ("error out"=w474:errorcluster, "ref out"=w503:i32, "value"=w475:dbl)  [unwired: 4 in]
                n282 = case shown="No Error" w474 {
                  tunnel: w475 -> [w530 _]
                  frame No Error {
                    "stop_time" <- w530
                  }
                  frame Error {
                  }
                }
                n283 = Build Array (concatenate)(w494, w493) -> (w492:u16[][][])
              }
              frame Error {
                n284 = Greater Than 0?(x=w536) -> (x > 0?=w535:bool)
                n285 = case shown="True" w535 {
                  tunnel: w534 -> [w539 _]
                  tunnel: [w539 w542] -> w533
                  frame False {
                  }
                  frame True {
                    n286 = local read "camera name"() -> (w540:string)
                    n287 = Concatenate Strings("Specified HDF has no instructions for camera " ("error message (\"\")"), w540) -> (w541:string)
                    n288 = call <vilib>:"Error Cluster From Error Code.vi"("error message (\"\")"=w541, "error code (0)"=6013) -> ("error out"=w542:errorcluster)  [unwired: 7 in]
                  }
                }
                n289 = local write "current file"("") -> ()
                n290 = property on="comp_data" class="Arr (strict)"() -> ("Value"=w531:T14)  [unwired: 2 in, 2 out]
                n291 = local read "sequencer"() -> (w537:T13)
                n292 = property on="image_data" class="Arr (strict)"() -> ("Value"=w532:u16[][][])  [unwired: 2 in, 2 out]
              }
            }
            "sequencer" <- w437
            n293 = call <vilib>:"H5F_close.vi"("error in (no error)"=w439, "ref"=w440) -> ("error out"=w418:errorcluster)  [unwired: 3 in]
            n294 = local write "image_data"(w438) -> ()
            n295 = local write "comp_data"(w435) -> ()
            n296 = for {
              tunnel: [w454] -> w436 mode=indexing
              tunnel: w435 -> [w452] mode=indexing
              n297 = Unbundle(w452) -> ("sequence"=w455:string, "name"=w453:string)  [unwired: 2 out]
              n298 = Build Array(w455, w453) -> (w454:string[])
            }
            n299 = case shown="Error" w418 {
              selector: w418 -> [_ w470]
              tunnel: [w469 w473] -> _
              tunnel: w451 -> [w469 w472]
              frame No Error {
              }
              frame Error {
                n300 = call <userlib>:"Notify_error.vi"("error in"=w470) -> ()  [unwired: 2 in, 1 out]
                n301 = local write "current file"("") -> ()
                n302 = Flush Queue(queue=w472) -> (queue out=w473:refnum<queue>)  [unwired: 1 in, 2 out]
              }
            }
            n303 = for {
              tunnel: w437 -> [w465] mode=indexing
              tunnel: [w462] -> w434 mode=indexing
              shift-right: [w459] -> w428
              shift-left: string[][] [] -> [w458]
              n304 = Unbundle(w465) -> ("name"=w460:string, "shots"=w461:string[])  [unwired: 1 out]
              n305 = Equal?(x=w460, y="(held)") -> (x = y?=w463:bool)
              n306 = for {
                tunnel: w461 -> [w468] mode=indexing
                tunnel: w460 -> [w467]
                tunnel: [w466] -> w457 mode=indexing
                n307 = Build Array(w467, w468) -> (w466:string[])
              }
              n308 = Boolean To (0,1)(Boolean=w463) -> (0, 1=w462:i16)
              n309 = Build Array (concatenate)(w457, w458) -> (w459:string[][])
            }
            n310 = call <vilib>:"Clear Errors.vi"("error in (no error)"=w418) -> ("error out"=w419:errorcluster)  [unwired: 6 in]
            n311 = Merge Errors(w416, w419) -> (w417:errorcluster)
            n312 = call <userlib>:"zlock_release.vi"("error in (no error)"=w417, "key"=w420, "ZLock in"=w421) -> ("error out"=w415:errorcluster)  [unwired: 6 in, 2 out]
            n313 = local write "fit_current"(FALSE ("fit_current")) -> ()
            n314 = Array Size(array=w435) -> (size(s)=w443:i32)
            n315 = property on="comp_list" class="MCListbox (strict)"("ItemNames"=w436) -> ()  [unwired: 2 in, 2 out]
            n316 = Greater Than 0?(x=w443) -> (x > 0?=w442:bool)
            n317 = case shown="True" w442 {
              frame False {
              }
              frame True {
                n318 = property on="comp_list" class="MCListbox (strict)"("Val(Sgnl)"=0 ("display_frame")) -> ()  [unwired: 2 in, 2 out]
              }
            }
            n319 = property on="n_atoms" class="DigNum (strict)"("DisabledEnum"=T22."Enabled" ("Disabled")) -> ()  [unwired: 2 in, 2 out]
            n320 = Add Array Elements(numeric array=w434) -> (sum=→"keep":i16)
            n321 = property on="raw_list" class="MCListbox (strict)"("ItemNames"=w428) -> ()  [unwired: 2 in, 2 out]
          }
          frame "" {
            n322 = call <userlib>:"BasicLogger.vi"("text"="Empty \"read file\" command") -> ()  [unwired: 6 in, 2 out]
          }
        }
      }
      frame "Save File" {
        n323 = local read "working dir"() -> (w549:path)
        n324 = local read "current file"() -> (w548:string)
        n325 = case shown="Default" w548 {
          selector: w548 -> [w568 _]
          tunnel: w549 -> [w569 _]
          tunnel: [w557 w634] -> w547
          tunnel: w546 -> [w554 _]
          tunnel: [w552 _] -> _
          frame Default {
            n326 = Build Path(base path=w569, name or relative path=w568) -> (appended path=w559:path)
            n327 = Path To String(path=w559) -> (string=w558:string)
            n328 = local read "location"() -> (w571:string)
            n329 = call <userlib>:"zlock_acquire.vi"("key"=w558, "ZLock in"=w554) -> ("error out"=w550:errorcluster, "key out"=w555:string, "ZLock out"=w553:T17)  [unwired: 7 in]
            n330 = Concatenate Strings("Save file  " ("text"), w568) -> (w572:string)
            n331 = call <vilib>:"H5F_open.vi"("error in (no error)"=w550, "mode"=H5F_mode."read-write", "path"=w559) -> ("error out"=w566:errorcluster, "ref"=w560:i32)  [unwired: 1 in]
            n332 = Concatenate Strings("images/" ("attribute"), w571) -> (w564:string)
            n333 = call <userlib>:"BasicLogger.vi"("text"=w572) -> ()  [unwired: 6 in, 2 out]
            n334 = call <vilib>:"H5G_open.vi"("error in (no error)"=w566, "create? (F)"=TRUE, "name"=w564, "ref"=w560) -> ("error out"=w565:errorcluster, "group"=w562:i32)  [unwired: 2 in]
            n335 = case shown="No Error" w565 {
              selector: w565 -> [_ w631]
              tunnel: [w582 w631] -> w561
              tunnel: w562 -> [w580 _]
              frame No Error {
                n336 = property on="rois" class="Arr (strict)"() -> ("Value"=w579:T7)  [unwired: 2 in, 2 out]
                n337 = local read "effective_pixel"() -> (w594:dbl)
                n338 = local read "camera name"() -> (w598:string)
                n339 = for {
                  tunnel: w580 -> [w609]
                  tunnel: w579 -> [w601] mode=indexing
                  tunnel: [w607] -> w578
                  shift-right: [w606] -> w577
                  shift-left: _ -> [w605]
                  i -> [w604]
                  n340 = Unbundle(w601) -> ("rect"=w600:T6)  [unwired: 3 out]
                  n341 = Format Into String(format string="roi%d", w604) -> (resulting string=w602:string)  [unwired: 2 in, 1 out]
                  n342 = call <userlib>:"Validate_Rect.vi"("rect"=w600) -> ("valid"=w599:bool)
                  n343 = case shown="True" w599 {
                    tunnel: w609 -> [w611 w618]
                    tunnel: TRUE ("overwrite? (F)") -> [_ w617]
                    tunnel: [w611 w616] -> w607
                    tunnel: [w610 w615] -> w606
                    tunnel: w605 -> [w610 w614]
                    tunnel: w602 -> [_ w613]
                    tunnel: w600 -> [_ w612]
                    frame False {
                    }
                    frame True {
                      n344 = call <vilib>:"H5A_write.vi"("value"=w612, "attrib_name"=w613, "error in (no error)"=w614, "overwrite? (F)"=w617, "ref"=w618) -> ("error out"=w615:errorcluster, "ref out"=w616:i32)  [unwired: 3 in]
                    }
                  }
                }
                n345 = local read "attribs"() -> (w596:variant[])
                n346 = call <userlib>:"Set Data Name__ogtk.vi"("Data Name"="effective_pixel_size", "Data"=w594) -> ("Renamed Data"=w592:variant)  [unwired: 8 in, 1 out]
                n347 = call <userlib>:"Set Data Name__ogtk.vi"("Data Name"="camera", "Data"=w598) -> ("Renamed Data"=w595:variant)  [unwired: 8 in, 1 out]
                n348 = Build Array (concatenate)(w592, w596, w595) -> (w591:variant[])
                n349 = property on="comp_data" class="Arr (strict)"() -> ("Value"=w574:T14)  [unwired: 2 in, 2 out]
                n350 = property on="image_data" class="Arr (strict)"() -> ("Value"=w576:u16[][][])  [unwired: 2 in, 2 out]
                n351 = call <vilib>:"H5A_write_multi.vi"("attribs"=w591, "overwrite?"=FALSE, "ref"=w578) -> ("error out"=w583:errorcluster, "ref out"=w587:i32)  [unwired: 5 in]
                n352 = property on="sequencer" class="Arr (strict)"() -> ("Value"=w575:T13)  [unwired: 2 in, 2 out]
                n353 = call <vilib>:"Clear Errors.vi"("error in (no error)"=w583) -> ()  [unwired: 6 in, 1 out]
                n354 = local read "fit_current"() -> (w581:bool)
                n355 = call <userlib>:"Write_raw_data.vi"("image_data"=w576, "sequencer"=w575, "ref in"=w587) -> ("error out"=w584:errorcluster, "ref out"=w588:i32)  [unwired: 3 in]
                n356 = call <userlib>:"Write_comp_data.vi"("comp_data"=w574, "ref in"=w588) -> ("error out"=w585:errorcluster, "ref out"=w589:i32)  [unwired: 2 in]
                n357 = case shown="True" w581 {
                  tunnel: w574 -> [_ w621]
                  tunnel: w589 -> [_ w620]
                  tunnel: [_ w619] -> w586
                  frame False {
                  }
                  frame True {
                    n358 = for {
                      tunnel: w621 -> [w630] mode=indexing
                      tunnel: w620 -> [w625]
                      tunnel: [w623] -> w619 mode=indexing
                      n359 = Unbundle By Name(w630) -> ("sequence"=w629:string, "name"=w628:string)
                      n360 = local read "fit_params"() -> (w622:T9)
                      n361 = local read "fit attribs"() -> (w626:variant[])
                      n362 = Concatenate Strings(w629, "/" ("string"), w628) -> (w624:string)
                      n363 = call <userlib>:"Write_fit_data.vi"("dset name"=w624, "fit attribs"=w626, "fit_params"=w622, "ref in"=w625) -> ("error out"=w623:errorcluster)  [unwired: 3 in, 1 out]
                    }
                  }
                }
                n364 = Merge Errors(w586, w585, w584, w577) -> (w582:errorcluster)
              }
              frame Error {
              }
            }
            n365 = call <vilib>:"H5F_close.vi"("error in (no error)"=w561, "ref"=w560) -> ("error out"=w557:errorcluster)  [unwired: 3 in]
            n366 = call <vilib>:"Clear Errors.vi"("error in (no error)"=w557) -> ("error out"=w556:errorcluster)  [unwired: 6 in]
            n367 = Merge Errors(w550, w556) -> (w551:errorcluster)
            n368 = call <userlib>:"zlock_release.vi"("error in (no error)"=w551, "key"=w555, "ZLock in"=w553) -> ("error out"=w552:errorcluster)  [unwired: 6 in, 2 out]
          }
          frame "" {
            n369 = call <vilib>:"Error Cluster From Error Code.vi"("error message (\"\")"="Cannot save file - no filename specified" ("error message (\"\")"), "error code (0)"=6015) -> ("error out"=w634:errorcluster)  [unwired: 7 in]
          }
        }
        n370 = call <userlib>:"Notify_error.vi"("error in"=w547) -> ()  [unwired: 2 in, 1 out]
      }
    }
  }
  n371 = while {
    tunnel: w21 -> [w636]
    tunnel: w54 -> [w637]
    stop <- FALSE stop-if-true
    n372 = event shown="[10] \"comp_ctrls\", \"raw_ctrls\": Value Change" {
      selector: _ -> [_ _ _ _ _ _ _ _ _ _ _ _ _ _ _ _ _ _]
      dyn-events: _ -> [_ _ _ _ _ _ _ _ _ _ _ _ _ _ _ _ _ _]
      timeout: 200 -> [_ _ _ _ _ _ _ _ _ _ _ _ _ _ _ _ _ _]
      tunnel: w637 -> [_ _ _ w670 w673 w716 _ _ w785 w805 _ _ _ _ _ _ _ _]
      tunnel: w636 -> [w639 _ _ _ _ w715 _ _ w784 _ _ _ w857 _ _ _ _ _]
      event Timeout {
        w641 = 4 items=["None", "Selection Tool", "Point Tool", "Line Tool", "Rectangle Tool", "Oval Tool", "Polygon Tool", "ClosedFreehandTool", "Annulus Tool", "Rotated Rectangle Tool", "Zoom Tool", "Pan Tool", "Polyline Tool", "Freehand Tool"] ("Tool")
        n373 = event-data() -> ()  [unwired: 1 in, 2 out]
        n374 = invoke on="img_OD" class="ImageControl" method="Get Last Event"("Which Events"=i32[] [2, 1]) -> ("Tool"=w642:i32)  [unwired: 7 in, 7 out]
        n375 = Equal?(x=w642, y=w641) -> (x = y?=w640:bool)
        n376 = case shown="True" w640 {
          tunnel: w639 -> [_ _]
          frame False {
          }
          frame True {
            n377 = property on="img_OD" class="ImageControl"() -> ("ROI"=w649:T32)  [unwired: 2 in, 2 out]
            n378 = call <userlib>:"ROI_to_rects.vi"("ROI"=w649) -> ("rect"=w648:T6)  [unwired: 3 out]
            n379 = local read "roi_capture"() -> (w647:T6)
            n380 = local read "roi_capture"() -> (w645:T6)
            n381 = call <userlib>:"Apply_Rect_Offset.vi"("offset rect"=w647, "input"=w648) -> ("output"=w646:T6)  [unwired: 3 in]
            n382 = call <userlib>:"Clip_Rect.vi"("bounds"=w645, "rect"=w646) -> ("result"=w644:T6)  [unwired: 1 in]
            n383 = property on="roi_current" class="Clust (strict)"("Val(Sgnl)"=w644) -> ()  [unwired: 2 in, 2 out]
          }
        }
      }
      event "newinst": Value Change {
        # "Doesn't appear to actually \"run\" the clone"
        n384 = event-data() -> ("NewVal"=w650:bool)  [unwired: 1 in, 4 out]
        n385 = case shown="True" w650 {
          tunnel: [_ w654] -> _
          frame False {
          }
          frame True {
            n386 = property class="VI"() -> ("Path"=w662:path)  [unwired: 2 in, 2 out]
            n387 = Open VI Reference(vi path=w662, options=8) -> (vi reference=w658:refnum<vi>)  [unwired: 4 in, 1 out]
            n388 = invoke class="VI" method="FP.Open"(reference=w658, "Activate"=TRUE ("Activate?"), "State"=T30."Maximized") -> (reference out=w660:refnum<vi>, error out=w659:errorcluster)  [unwired: 2 in, 3 out]
            n389 = invoke class="VI" method="Run VI"(reference=w660, error in=w659, "Wait until done"=FALSE ("Wait Until Done")) -> (reference out=w656:refnum<vi>, error out=w657:errorcluster)  [unwired: 2 in, 3 out]
            n390 = local write "newinst"(FALSE ("newinst")) -> ()
            n391 = Close Reference(reference=w656, error in (no error)=w657) -> (error out=w654:errorcluster)
          }
        }
      }
      event Value Change {
        # "Something with interrupts to improve flicker"
        n392 = event-data() -> ()  [unwired: 1 in, 5 out]
        n393 = local read "roi_capture"() -> (w667:T6)
        n394 = local read "roi_current"() -> (w663:T6)
        n395 = Negate(x=w667) -> (-x=w666:T6)
        n396 = call <userlib>:"Apply_Rect_Offset.vi"("offset rect"=w666, "input"=w663) -> ("output"=w665:T6)  [unwired: 3 in]
        n397 = call <userlib>:"Rect_to_ROI.vi"("rect"=w665) -> ("ROI"=w664:T33)
        n398 = property on="img_OD" class="ImageControl"("ROI"=w664) -> ()  [unwired: 2 in, 2 out]
      }
      event "stop": Value Change {
        n399 = event-data() -> ()  [unwired: 1 in, 5 out]
        n400 = Flush Queue(queue=w670) -> (queue out=w668:refnum<queue>)  [unwired: 1 in, 2 out]
        n401 = Enqueue Element(queue=w668, element=Imaging_State."Quit") -> ()  [unwired: 2 in, 3 out]
      }
      event "files": Value Change {
        n402 = event-data() -> ("OldVal"=w675:T1, "NewVal"=w674:T1)  [unwired: 1 in, 3 out]
        n403 = Cluster To Array(cluster=w675) -> (array=w677:bool[])
        n404 = Cluster To Array(cluster=w674) -> (array=w676:bool[])
        n405 = call <userlib>:"Detect_Boolean_Change.vi"("NewVal"=w676, "OldVal"=w677) -> ("ButtonId"=w672:i32)  [unwired: 2 out]
        n406 = Greater Or Equal To 0?(x=w672) -> (x >= 0?=w671:bool)
        n407 = case shown="True" w671 {
          tunnel: w673 -> [_ w678]
          tunnel: w672 -> [_ w679]
          frame False {
          }
          frame True {
            n408 = local read "current file"() -> (w680:string)
            n409 = case shown="0, 1" w679 {
              selector: w679 -> [_ _ _ w687]
              tunnel: w680 -> [_ _ _ w695]
              tunnel: w678 -> [w681 w683 _ w688]
              frame 2 {
                n410 = Enqueue Element(queue=w681, element=Imaging_State."Save File") -> ()  [unwired: 2 in, 3 out]
              }
              frame 3 {
                n411 = Enqueue Element(queue=w683, element=Imaging_State."Compute") -> ()  [unwired: 2 in, 3 out]
              }
              frame Default {
              }
              frame 0, 1 {
                n412 = local read "working dir"() -> (w692:path)
                n413 = call "File Dialog"("start path"=w692, "prompt"="Select H5 File", "default name"=w695, "pattern (all files)"="*.h5", "pattern label"="HDF files") -> ("selected path"=w693:path, "error out"=w686:errorcluster)  [unwired: 7 in, 2 out]
                n414 = call <vilib>:"H5F_is_hdf.vi"("error in (no error)"=w686, "path"=w693) -> ("error out"=w685:errorcluster, "valid"=w694:bool)  [unwired: 1 in, 1 out]
                n415 = case shown="False" w694 {
                  tunnel: w693 -> [_ w708]
                  tunnel: w688 -> [_ w707]
                  tunnel: w687 -> [_ w697]
                  tunnel: w685 -> [_ _]
                  frame False {
                    n416 = One Button Dialog(message="Chosen file is not a valid HDF5") -> ()  [unwired: 1 in, 1 out]
                  }
                  frame True {
                    n417 = Flush Queue(queue=w707) -> (queue out=w703:refnum<queue>, remaining elements=w706:T11[])  [unwired: 1 in, 1 out]
                    n418 = Strip Path(path=w708) -> (stripped path=w705:path, name=w704:string)
                    n419 = property on="working dir" class="Path"("Value"=w705) -> (error out=w700:errorcluster)  [unwired: 2 in, 1 out]
                    n420 = Array Size(array=w706) -> (size(s)=w698:i32)
                    n421 = property on="current file" class="Str"(error in=w700, "Value"=w704) -> (error out=w699:errorcluster)  [unwired: 1 in, 1 out]
                    n422 = Enqueue Element(queue=w703, element=Imaging_State."Read File", error in (no error)=w699) -> (queue out=w701:refnum<queue>)  [unwired: 1 in, 2 out]
                    n423 = case shown="Default" w698 {
                      frame 0 {
                      }
                      frame Default {
                        n424 = call <userlib>:"BasicLogger.vi"("text"="File open forced queue clear") -> ()  [unwired: 6 in, 2 out]
                      }
                    }
                    n425 = case shown="Default" w697 {
                      tunnel: w701 -> [w711 w712]
                      frame Default {
                        n426 = Enqueue Element(queue=w711, element=Imaging_State."Redraw") -> ()  [unwired: 2 in, 3 out]
                      }
                      frame 1 {
                        n427 = Enqueue Element(queue=w712, element=Imaging_State."Acquire") -> ()  [unwired: 2 in, 3 out]
                      }
                    }
                  }
                }
              }
            }
          }
        }
      }
      event "capture.abort": Value Change {
        n428 = event-data() -> ("NewVal"=w714:bool)  [unwired: 1 in, 4 out]
        n429 = case shown="True" w714 {
          tunnel: w716 -> [_ w721]
          tunnel: w715 -> [_ w720]
          tunnel: [_ w717] -> _
          frame False {
          }
          frame True {
            n430 = Flush Queue(queue=w721) -> (error out=w718:errorcluster)  [unwired: 1 in, 2 out]
            n431 = call-dynamic "CameraAbort.vi"("error in (no error)"=w718, "CameraBase in"=w720) -> ("error out"=w717:errorcluster)  [unwired: 8 in, 1 out]
            n432 = call <userlib>:"BasicLogger.vi"("text"="Abort signalled") -> ()  [unwired: 6 in, 2 out]
          }
        }
      }
      event "tools_zoom": Value Change {
        n433 = event-data() -> ("OldVal"=w725:T2, "NewVal"=w724:T2)  [unwired: 1 in, 3 out]
        n434 = control-ref of="img_OD"() -> (w722:refnum<vi>)
        n435 = Cluster To Array(cluster=w725) -> (array=w726:bool[])
        n436 = Cluster To Array(cluster=w724) -> (array=w727:bool[])
        n437 = call <userlib>:"Detect_Boolean_Change.vi"("NewVal"=w727, "OldVal"=w726) -> ("ButtonId"=w728:i32)  [unwired: 2 out]
        n438 = Build Array(w722) -> (w723:refnum<vi>[])
        n439 = for {
          tunnel: w728 -> [w730]
          tunnel: [w729] -> _ mode=indexing
          tunnel: w723 -> [w729] mode=indexing
          n440 = case shown="0" w730 {
            tunnel: w729 -> [w731 w748 w760 w768 _]
            frame 0 {
              n441 = property on="Property Node" class="ImageControl" props=["ROI", "Image Area Size", "Image Area Height", "Image Area Width"](reference=w731) -> (reference out=w732:refnum<vi>, "ROI"=w738:T32, "Image Area Height"=w737:u32, "Image Area Width"=w736:u32)  [unwired: 1 in, 2 out]
              n442 = Unbundle(w738) -> ("Global Rectangle"=w735:i32[], "Contours"=w734:T34)
              n443 = Empty Array?(array=w734) -> (empty?=w733:bool)
              n444 = case shown="False" w733 {
                tunnel: w737 -> [w747 _]
                tunnel: w736 -> [w746 _]
                tunnel: w735 -> [w743 _]
                tunnel: w732 -> [w739 _]
                frame False {
                  n445 = formula code="Zx=W/(R[2]-R[0]);\nZy=H/(R[3]-R[1]);\nCx=(R[2]+R[0])/2;\nCy=(R[3]+R[1])/2;"("R"=w743, "H"=w747, "W"=w746) -> ("Zx"=w741:dbl, "Zy"=w742:dbl, "Cx"=w745:dbl, "Cy"=w744:dbl)
                  n446 = Max & Min(x=w741, y=w742) -> (min(x,y)=w740:dbl)  [unwired: 1 out]
                  n447 = property on="Property Node" class="ImageControl"(reference=w739, "X Zoom"=w740, "Y Zoom"=w740, "Image Center X Position"=w745, "Image Center Y Position"=w744) -> ()  [unwired: 1 in, 2 out]
                }
                frame True {
                }
              }
            }
            frame 1 {
              w755 = sgl 1.2 ("x")
              # "Zoom to ROI if possible"
              n448 = property on="Property Node" class="ImageControl"(reference=w748) -> (reference out=w749:refnum<vi>, "X Zoom"=w756:sgl, "Y Zoom"=w757:sgl, "ROI"=w754:T32, "Image Center Position"=w750:cluster{"X":u32, "Y":u32})  [unwired: 1 in, 1 out]
              n449 = call <userlib>:"ROI_to_rects.vi"("ROI"=w754) -> ("center"=w752:cluster{"x":i16, "y":i16}, "valid"=w753:bool)  [unwired: 2 out]
              n450 = Select(t=w752, s=w753, f=w750) -> (s? t:f=w751:cluster{"X":u32, "Y":u32})
              n451 = Multiply(x=w756, y=w755) -> (x*y=w759:sgl)
              n452 = Multiply(x=w757, y=w755) -> (x*y=w758:sgl)
              n453 = property on="Property Node" class="ImageControl"(reference=w749, "X Zoom"=w759, "Y Zoom"=w758, "Image Center Position"=w751) -> ()  [unwired: 1 in, 2 out]
            }
            frame 2 {
              w762 = sgl 1.2 ("x")
              n454 = property on="Property Node" class="ImageControl"(reference=w760) -> (reference out=w761:refnum<vi>, "X Zoom"=w764:sgl, "Y Zoom"=w765:sgl, "Image Center Position"=w763:cluster{"X":u32, "Y":u32})  [unwired: 1 in, 1 out]
              n455 = Divide(x=w764, y=w762) -> (x/y=w767:sgl)
              n456 = Divide(x=w765, y=w762) -> (x/y=w766:sgl)
              n457 = property on="Property Node" class="ImageControl"(reference=w761, "X Zoom"=w767, "Y Zoom"=w766, "Image Center Position"=w763) -> ()  [unwired: 1 in, 2 out]
            }
            frame 3 {
              n458 = property on="Property Node" class="ImageControl"(reference=w768, "Zoom to Fit Mode"=TRUE) -> ()  [unwired: 1 in, 2 out]
            }
            frame Default {
            }
          }
        }
      }
      event "tools_view": Value Change {
        n459 = event-data() -> ("OldVal"=w772:cluster{"sel":bool, "in":bool, "out":bool}, "NewVal"=w771:cluster{"sel":bool, "in":bool, "out":bool})  [unwired: 1 in, 3 out]
        n460 = Cluster To Array(cluster=w772) -> (array=w779:bool[])
        n461 = Cluster To Array(cluster=w771) -> (array=w778:bool[])
        n462 = call <userlib>:"Detect_Boolean_Change.vi"("NewVal"=w778, "OldVal"=w779) -> ("FinalVal"=w776:bool[], "SingleEvent"=w774:bool, "ButtonId"=w777:i32)
        n463 = Array To Cluster(array=w776) -> (cluster=w773:T35)
        n464 = Select(t=w773, s=w774, f=w772) -> (s? t:f=w770:cluster{"sel":bool, "in":bool, "out":bool})
        n465 = case shown="0" w777 {
          tunnel: [w780 w781 w782 w783] -> w775
          frame Default {
            n466 = property on="img_OD" class="ImageControl"() -> ("Current ROI Tool"=w780:u32)  [unwired: 2 in, 2 out]
          }
          frame 0 {
            w781 = u32 8 items=["No Selection", "Point", "Line", "Rectangle", "Oval", "Polygon", "Freehand Region", "Annulus", "Zoom", "Pan", "Broken Line", "Freehand Line", "Rotated Rectangle"] ("Tool (Point)")
          }
          frame 1 {
            w782 = u32 3 items=["No Selection", "Point", "Line", "Rectangle", "Oval", "Polygon", "Freehand Region", "Annulus", "Zoom", "Pan", "Broken Line", "Freehand Line", "Rotated Rectangle"] ("Tool (Point)")
          }
          frame 2 {
            w783 = u32 9 items=["No Selection", "Point", "Line", "Rectangle", "Oval", "Polygon", "Freehand Region", "Annulus", "Zoom", "Pan", "Broken Line", "Freehand Line", "Rotated Rectangle"] ("Tool (Point)")
          }
        }
        n467 = local write "tools_view"(w770) -> ()
        n468 = property on="img_OD" class="ImageControl"("Current ROI Tool"=w775) -> ()  [unwired: 2 in, 2 out]
      }
      event "capture": Value Change {
        n469 = event-data() -> ("OldVal"=w786:T3, "NewVal"=w787:T3)  [unwired: 1 in, 3 out]
        n470 = Cluster To Array(cluster=w786) -> (array=w790:bool[])
        n471 = Cluster To Array(cluster=w787) -> (array=w789:bool[])
        n472 = call <userlib>:"Detect_Boolean_Change.vi"("NewVal"=w789, "OldVal"=w790) -> ("ButtonId"=w788:i32)  [unwired: 2 out]
        n473 = case shown="0, 1" w788 {
          selector: w788 -> [w799 _]
          tunnel: w785 -> [w795 _]
          tunnel: w784 -> [w793 _]
          frame 0, 1 {
            n474 = local read "roi_current"() -> (w801:T6)
            n475 = local read "roi_sensor"() -> (w798:T6)
            n476 = Equal To 0?(x=w799) -> (x = 0?=w800:bool)
            n477 = call <userlib>:"Validate_Rect_Default.vi"("rect"=w801, "default"=w798) -> ("out"=w797:T6)
            n478 = Select(t=w797, s=w800, f=w798) -> (s? t:f=w792:T6)
            n479 = call-dynamic "CameraCheckROI.vi"("ROI_in"=w792, "CameraBase in"=w793) -> ("ROI_out"=w791:T6)  [unwired: 7 in, 2 out]
            n480 = property on="roi_capture" class="Clust (strict)"("Val(Sgnl)"=w791) -> (error out=w794:errorcluster)  [unwired: 2 in, 1 out]
            n481 = Enqueue Element(queue=w795, element=Imaging_State."Software trigger", error in (no error)=w794) -> ()  [unwired: 1 in, 3 out]
          }
          frame Default {
          }
        }
      }
      event "fit_buttons": Value Change {
        # "redraw ROIs"
        n482 = event-data() -> ("OldVal"=w808:cluster{"selection":bool, "stored":bool}, "NewVal"=w809:cluster{"selection":bool, "stored":bool})  [unwired: 1 in, 3 out]
        n483 = Cluster To Array(cluster=w808) -> (array=w810:bool[])
        n484 = Cluster To Array(cluster=w809) -> (array=w811:bool[])
        n485 = call <userlib>:"Detect_Boolean_Change.vi"("NewVal"=w811, "OldVal"=w810) -> ("ButtonId"=w806:i32)  [unwired: 2 out]
        n486 = case shown="0" w806 {
          tunnel: [_ w812] -> w803
          frame Default {
          }
          frame 0 {
            n487 = local read "roi_current"() -> (w814:T6)
            n488 = local read "fit_roi"() -> (w815:T10)
            n489 = Bundle By Name(cluster=w815, "rect"=w814) -> (w813:T10)
            n490 = property on="fit_roi" class="Clust (strict)"("Value"=w813) -> (error out=w812:errorcluster)  [unwired: 2 in, 1 out]
          }
        }
        n491 = local read "rois"() -> (w804:T7)
        n492 = property on="rois" class="Arr (strict)"(error in=w803, "Val(Sgnl)"=w804) -> (error out=w802:errorcluster)  [unwired: 1 in, 1 out]
        n493 = Enqueue Element(queue=w805, element=Imaging_State."Fit", error in (no error)=w802) -> ()  [unwired: 1 in, 3 out]
      }
      event Value Change {
        n494 = event-data() -> ("CtlRef"=w822:refnum<vi>, "OldVal"=w819:T8, "NewVal"=w818:T8)  [unwired: 1 in, 2 out]
        n495 = Unbundle By Name(w818) -> ("val_max"=w821:sgl)
        n496 = Unbundle By Name(w819) -> ("val_max"=w820:sgl)
        n497 = Not Equal?(x=w821, y=w820) -> (x != y?=w823:bool)
        n498 = case shown="True" w823 {
          tunnel: w822 -> [_ w826]
          tunnel: [_ w827] -> w816
          tunnel: w818 -> [_ w824]
          frame False {
          }
          frame True {
            n499 = Bundle By Name(cluster=w824, "automax"=FALSE) -> (w825:T8)
            n500 = property class="Clust (strict)"(reference=w826, "Value"=w825) -> (error out=w827:errorcluster)  [unwired: 1 in, 1 out]
          }
        }
        n501 = local read "frame"() -> (w817:i32)
        n502 = property on="frame" class="DigNum (strict)"(error in=w816, "Val(Sgnl)"=w817) -> ()  [unwired: 1 in, 2 out]
      }
      event Value Change {
        n503 = event-data() -> ("CtlRef"=w829:refnum<vi>, "NewVal"=w833:u16)  [unwired: 1 in, 3 out]
        n504 = property class="Ring (strict)"(reference=w829) -> ("Owner"=w835:refnum<vi>)  [unwired: 1 in, 2 out]
        n505 = local read "frame"() -> (w836:i32)
        n506 = control-ref of="raw_ctrls"() -> (w834:refnum<vi>)
        n507 = Equal?(x=w835, y=w834) -> (x = y?=w832:bool)
        n508 = Greater Or Equal To 0?(x=w836) -> (x >= 0?=w831:bool)
        n509 = Not Exclusive Or(1:w831, 2:w832) -> (0:w830:bool)
        n510 = case shown="True" w830 {
          tunnel: w833 -> [_ w840]
          tunnel: w829 -> [_ w837]
          frame False {
          }
          frame True {
            n511 = case shown="Default" w840 {
              tunnel: [w844 w852 w853 w854 w856] -> w839
              tunnel: [w843 _ _ _ w855] -> w838
              tunnel: w837 -> [w842 _ _ _ _]
              frame Default {
                w844 = u32 5 items=["Grayscale", "Binary", "Gradient", "Rainbow", "Temperature", "User Defined"] ("Palette:Palette Type")
                n512 = property on="Property Node" class="Ring (strict)"(reference=w842) -> ("RingText.Text"=w841:string)  [unwired: 1 in, 2 out]
                n513 = Concatenate Strings(w841, ".tsv" ("string")) -> (w845:string)
                n514 = Build Path(base path=path "Z:/Temp/rgb gradients", name or relative path=w845) -> (appended path=w848:path)
                n515 = call-poly <vilib>:"Read From Spreadsheet File.vi"("file path (dialog if empty)"=w848) -> ("all rows"=w849:dbl[][])  [unwired: 6 in, 4 out]
                n516 = for {
                  tunnel: w849 -> [w851] mode=indexing
                  tunnel: [w850] -> w843 mode=indexing
                  n517 = Array To Cluster(array=w851) -> (cluster=w850:T36)
                }
              }
              frame 0 {
                w852 = u32 0 items=["Grayscale", "Binary", "Gradient", "Rainbow", "Temperature", "User Defined"] ("Palette:Palette Type")
              }
              frame 1 {
                w853 = u32 3 items=["Grayscale", "Binary", "Gradient", "Rainbow", "Temperature", "User Defined"] ("Palette:Palette Type")
              }
              frame 2 {
                w854 = u32 4 items=["Grayscale", "Binary", "Gradient", "Rainbow", "Temperature", "User Defined"] ("Palette:Palette Type")
              }
              frame 3 {
                n518 = property on="img_OD" class="ImageControl"() -> ("Palette Type"=w856:u32, "User Palette"=w855:cluster{"Red":u8, "Green":u8, "Blue":u8}[])  [unwired: 2 in, 2 out]
              }
            }
            n519 = property on="img_OD" class="ImageControl"("Palette Type"=w839, "User Palette"=w838) -> ()  [unwired: 2 in, 2 out]
          }
        }
      }
      event "config_cam": Mouse Up {
        n520 = event-data() -> ()  [unwired: 1 in, 8 out]
        n521 = call-dynamic "CameraSetProperties.vi"("set?"=TRUE, "CameraBase in"=w857) -> ("cam_params"=w858:cluster{"String":string, "value":variant}[])  [unwired: 7 in, 2 out]
        n522 = local write "cam_params"(w858) -> ()
      }
      event "last error.status": Value Change; "last error.status", "recent_error": Mouse Up {
        n523 = event-data() -> ("Type"=w864:T31, "CtlRef"=w860:refnum<vi>)  [unwired: 1 in, 2 out]
        n524 = Equal?(x=lveventtype."Mouse Up" ("Type"), y=w864) -> (x = y?=w862:bool)
        n525 = case shown="False" w862 {
          tunnel: [w866 FALSE ("recent_error")] -> w861
          tunnel: w860 -> [w865 _]
          frame False {
            n526 = property on="Property Node" class="Bool (strict)"(reference=w865) -> ("Value"=w866:bool)  [unwired: 1 in, 2 out]
          }
          frame True {
          }
        }
        "recent_error" <- w861
      }
      event "raw_list", "comp_list": Value Change {
        n527 = event-data() -> ("CtlRef"=w875:refnum<vi>, "OldVal"=w873:i32, "NewVal"=w874:i32)  [unwired: 1 in, 2 out]
        n528 = Greater Or Equal To 0?(x=w873) -> (x >= 0?=w872:bool)
        n529 = Not Equal?(x=w873, y=w874) -> (x != y?=w877:bool)
        n530 = Greater Or Equal To 0?(x=w874) -> (x >= 0?=w871:bool)
        n531 = And(x=w877, y=w871) -> (x .and. y?=w876:bool)
        n532 = Exclusive Or(1:w872, 2:w871) -> (0:w870:bool)
        n533 = case shown="True" w876 {
          tunnel: w875 -> [_ w889]
          tunnel: w874 -> [_ w888]
          tunnel: w870 -> [_ w881]
          tunnel: [_ w880] -> w869
          tunnel: [w878 w879] -> w868
          frame False {
            n534 = local read "frame"() -> (w878:i32)
          }
          frame True {
            # "Set the other one to -1"
            n535 = control-ref of="raw_list"() -> (w885:refnum<vi>)
            n536 = Equal?(x=w885, y=w889) -> (x = y?=w882:bool)
            n537 = Negate(x=w888) -> (-x=w890:i32)
            n538 = Decrement(x=w890) -> (x-1=w887:i32)
            n539 = Select(t=w888, s=w882, f=w887) -> (s? t:f=w879:i32)
            n540 = control-ref of="comp_list"() -> (w886:refnum<vi>)
            n541 = case shown="True" w881 {
              tunnel: w882 -> [_ w897]
              frame False {
              }
              frame True {
                n542 = control-ref of="col_scheme"() -> (w895:refnum<vi>)
                n543 = control-ref of="col_scheme"() -> (w896:refnum<vi>)
                n544 = Select(t=w896, s=w897, f=w895) -> (s? t:f=w894:refnum<vi>)
                n545 = property class="Ring (strict)"(reference=w894) -> (reference out=w893:refnum<vi>, error out=w892:errorcluster, "Value"=w891:u16)  [unwired: 1 in]
                n546 = property class="Ring (strict)"(reference=w893, error in=w892, "Val(Sgnl)"=w891) -> ()  [unwired: 2 out]
              }
            }
            n547 = Select(t=w886, s=w882, f=w885) -> (s? t:f=w884:refnum<vi>)
            n548 = property class="MCListbox (strict)"(reference=w884, "Value"=-1) -> (error out=w880:errorcluster)  [unwired: 1 in, 1 out]
          }
        }
        n549 = property on="frame" class="DigNum (strict)"(error in=w869, "Val(Sgnl)"=w868) -> ()  [unwired: 1 in, 2 out]
      }
      event "fit_roi": Value Change {
        w902 = FALSE ("get")
        # "redraw ROIs"
        n550 = event-data() -> ("CtlRef"=w900:refnum<vi>, "NewVal"=w904:T10)  [unwired: 1 in, 3 out]
        n551 = Unbundle(w904) -> ("get"=w909:bool, "set"=w908:bool, "rect"=w905:T6)  [unwired: 1 out]
        n552 = Build Array(w909, w908) -> (w907:bool[])
        n553 = Boolean Array To Number(Boolean array=w907) -> (number=w906:u32)
        n554 = case shown="2" w906 {
          tunnel: w905 -> [w910 _ w912]
          tunnel: [w910 w911 w912] -> w903
          frame Default {
          }
          frame 1 {
            n555 = local read "roi_current"() -> (w911:T6)
          }
          frame 2 {
            n556 = property on="roi_current" class="Clust (strict)"("Val(Sgnl)"=w912) -> ()  [unwired: 2 in, 2 out]
          }
        }
        n557 = Bundle(cluster=w904, "get"=w902, "set"=w902, "rect"=w903) -> (w901:T10)  [unwired: 1 in]
        n558 = property class="Clust (strict)"(reference=w900, "Value"=w901) -> (error out=w898:errorcluster)  [unwired: 1 in, 1 out]
        n559 = local read "rois"() -> (w899:T7)
        n560 = property on="rois" class="Arr (strict)"(error in=w898, "Val(Sgnl)"=w899) -> ()  [unwired: 1 in, 2 out]
      }
      event "rois": Value Change {
        n561 = event-data() -> ("CtlRef"=w914:refnum<vi>, "NewVal"=w916:T7)  [unwired: 1 in, 3 out]
        n562 = for {
          tunnel: w916 -> [w953] mode=indexing
          tunnel: [w950] -> w915 mode=indexing
          w951 = FALSE ("get")
          n563 = Unbundle(w953) -> ("get"=w958:bool, "set"=w957:bool, "rect"=w954:T6)  [unwired: 1 out]
          n564 = Build Array(w958, w957) -> (w956:bool[])
          n565 = Boolean Array To Number(Boolean array=w956) -> (number=w955:u32)
          n566 = case shown="1" w955 {
            tunnel: w954 -> [w959 _ w961]
            tunnel: [w959 w960 w961] -> w952
            frame Default {
            }
            frame 1 {
              # "set using roi_current"
              n567 = local read "roi_current"() -> (w960:T6)
            }
            frame 2 {
              n568 = property on="roi_current" class="Clust (strict)"("Val(Sgnl)"=w961) -> ()  [unwired: 2 in, 2 out]
            }
          }
          n569 = Bundle(cluster=w953, "get"=w951, "set"=w951, "rect"=w952) -> (w950:T10)  [unwired: 1 in]
        }
        n570 = property class="Arr (strict)"(reference=w914, "Value"=w915) -> (error out=w913:errorcluster)  [unwired: 1 in, 1 out]
        n571 = flat-sequence {
          tunnel: w913 -> [_]
          frame #0 {
            n572 = local read "img_OD"() -> (w920:T4)
            n573 = call "IMAQ Clear Overlay"("Groups"=string[] ["roi"], "Image"=w920) -> ("error out"=w924:errorcluster, "Image Out"=w922:T4)  [unwired: 8 in]
            n574 = call <vilib>:"Clear Errors.vi"("error in (no error)"=w924) -> ()  [unwired: 6 in, 1 out]
            n575 = local read "roi_capture"() -> (w925:T6)
            n576 = Build Array (concatenate)("rois", "fit_roi") -> (w919:T7)
            n577 = Negate(x=w925) -> (-x=w926:T6)
            n578 = local read "bin_x"() -> (w927:u8)
            n579 = local read "bin_y"() -> (w928:u8)
            n580 = Bundle("bin_x"=w927, "bin_y"=w928, "bin_x"=w927, "bin_y"=w928) -> (w929:T37)  [unwired: 1 in]
            n581 = for {
              tunnel: w919 -> [w937] mode=indexing
              shift-right: [w934] -> w923
              shift-left: w922 -> [w938]
              tunnel: w926 -> [w931]
              tunnel: w929 -> [w930]
              n582 = Unbundle By Name(w937) -> ("color"=w935:u32, "rect"=w932:T6)
              n583 = Not Equal?(x=u32 16777216, y=w935) -> (x != y?=w933:bool)
              n584 = case shown="True" w933 {
                tunnel: w938 -> [w939 w949]
                tunnel: w935 -> [_ w947]
                tunnel: [w939 w946] -> w934
                tunnel: w932 -> [_ w945]
                tunnel: w931 -> [_ w944]
                tunnel: w930 -> [_ w942]
                frame False {
                }
                frame True {
                  n585 = call <userlib>:"Apply_Rect_Offset.vi"("offset rect"=w944, "input"=w945) -> ("output"=w943:T6)  [unwired: 3 in]
                  n586 = Divide(x=w943, y=w942) -> (x/y=w941:cluster{dbl, dbl, dbl, dbl})
                  n587 = To Long Integer(number=w941) -> (32bit integer=w940:cluster{i32, i32, i32, i32})
                  n588 = call "IMAQ Overlay Rectangle"("Color"=w947, "Group"="roi", "Rectangle"=w940, "Image"=w949) -> ("Image Out"=w946:T4)  [unwired: 6 in, 1 out]
                }
              }
            }
            n589 = local write "img_OD"(w923) -> ()
          }
        }
      }
      event "frame": Value Change {
        # "redraw ROIs"
        # "Manually rescale to an I16"
        # "We've changed type, so switch color schemes"
        # "Do we actually have the frame we're supposed to show?"
        n590 = event-data() -> ("NewVal"=w968:i32)  [unwired: 1 in]
        n591 = property on="image_data" class="Arr (strict)"() -> ("Value"=w963:u16[][][])  [unwired: 2 in, 2 out]
        n592 = property on="comp_data" class="Arr (strict)"() -> ("Value"=w964:T14)  [unwired: 2 in, 2 out]
        n593 = Less Than 0?(x=w968) -> (x < 0?=w984:bool)
        n594 = case shown="True" w984 {
          tunnel: w968 -> [w994 w1001]
          tunnel: w964 -> [_ w1004]
          tunnel: [w992 w999] -> w987
          tunnel: w963 -> [w998 _]
          frame False {
            n595 = Array Size(array=w998) -> (size(s)=w997:i32[])
            n596 = Index Array(array=w997) -> (element=w996:i32)  [unwired: 1 in]
            n597 = Less?(x=w994, y=w996) -> (x < y?=w995:bool)
            n598 = Select(t=w994, s=w995, f=0) -> (s? t:f=w992:i32)
          }
          frame True {
            n599 = Negate(x=w1001) -> (-x=w1003:i32)
            n600 = Array Size(array=w1004) -> (size(s)=w1005:i32)
            n601 = Less Or Equal?(x=w1003, y=w1005) -> (x <= y?=w1002:bool)
            n602 = Select(t=w1001, s=w1002, f=0) -> (s? t:f=w999:i32)
          }
        }
        n603 = Less Than 0?(x=w987) -> (x < 0?=w983:bool)
        n604 = local write "frame"(w987) -> ()
        n605 = case shown="True" w983 {
          tunnel: [w1010 w1013] -> w976
          tunnel: w987 -> [w1008 w1017]
          tunnel: [w1009 w1014] -> w979
          tunnel: w964 -> [_ w1012]
          tunnel: w963 -> [w1007 _]
          tunnel: [w1006 w1011] -> w986
          frame False {
            # "RAW DATA"
            n606 = Index Array(array=w1007, index (dim 0)=w1008) -> (element=w1010:u16[][])  [unwired: 2 in]
            n607 = control-ref of="col_scheme"() -> (w1006:refnum<vi>)
            n608 = control-ref of="raw_ctrls"() -> (w1009:refnum<vi>)
          }
          frame True {
            # "COMPUTED DATA"
            n609 = Increment(x=w1017) -> (x+1=w1016:i32)
            n610 = Negate(x=w1016) -> (-x=w1015:i32)
            n611 = Index Array(array=w1012, index=w1015) -> (element=w1018:T25)
            n612 = control-ref of="col_scheme"() -> (w1011:refnum<vi>)
            n613 = control-ref of="comp_ctrls"() -> (w1014:refnum<vi>)
            n614 = Unbundle By Name(w1018) -> ("data"=w1013:sgl[][])
          }
        }
        n615 = Exclusive Or(1:w984, 2:w983) -> (0:w985:bool)
        n616 = case shown="True" w985 {
          tunnel: w986 -> [_ w991]
          frame False {
          }
          frame True {
            n617 = property class="Ring (strict)"(reference=w991) -> (reference out=w990:refnum<vi>, error out=w988:errorcluster, "Value"=w989:u16)  [unwired: 1 in]
            n618 = property class="Ring (strict)"(reference=w990, error in=w988, "Val(Sgnl)"=w989) -> ()  [unwired: 2 out]
          }
        }
        n619 = property class="Clust (strict)"(reference=w979) -> (reference out=w977:refnum<vi>, "Value"=w980:T8)  [unwired: 1 in, 1 out]
        n620 = Unbundle By Name(w980) -> ("automax"=w982:bool, "val_max"=w978:sgl, "val_min"=w981:sgl)
        n621 = Subtract(x=w976, y=w981) -> (x-y=w973:sgl[][])
        n622 = case shown="True" w982 {
          tunnel: [w1019 w1022] -> w969
          tunnel: w976 -> [_ w1024]
          tunnel: w977 -> [_ w1023]
          tunnel: w978 -> [w1019 _]
          tunnel: w980 -> [_ w1020]
          frame False {
          }
          frame True {
            # "Recompute maximum value"
            n623 = Array Max & Min(array=w1024) -> (max value=w1022:sgl)  [unwired: 3 out]
            n624 = Bundle By Name(cluster=w1020, "val_max"=w1022) -> (w1021:T8)
            n625 = property class="Clust (strict)"(reference=w1023, "Value"=w1021) -> ()  [unwired: 1 in, 2 out]
          }
        }
        n626 = Subtract(x=w969, y=w981) -> (x-y=w970:sgl)
        n627 = Divide(x=32767.0, y=w970) -> (x/y=w972:dbl)
        n628 = Multiply(x=w973, y=w972) -> (x*y=w974:dbl[][])
        n629 = local read "img_OD"() -> (w965:T4)
        n630 = To Word Integer(number=w974) -> (16bit integer=w962:i16[][])
        n631 = local read "rois"() -> (w967:T7)
        n632 = call "IMAQ ArrayToImage"("Image Pixels (I16)"=w962, "Image"=w965) -> ("error out"=w966:errorcluster, "Image Out"=w975:T4)  [unwired: 8 in]
        n633 = local write "img_OD"(w975) -> ()
        n634 = property on="rois" class="Arr (strict)"(error in=w966, "Val(Sgnl)"=w967) -> ()  [unwired: 1 in, 2 out]
      }
    }
  }
  n635 = while {
    tunnel: w53 -> [w1032]
    tunnel: w21 -> [w1025]
    tunnel: w54 -> [w1027]
    stop <- FALSE stop-if-true
    # "Wait for TCP"
    # "Run forever"
    n636 = TCP Wait On Listener(11:w1032) -> (0:w1029:errorcluster, 1:w1030:u16, 2:w1031:string, 4:w1026:refnum<k5>)  [unwired: 3 in, 1 out]
    n637 = Format Into String(format string=":%d", initial string=w1031, w1030) -> (resulting string=w1033:string)  [unwired: 1 in, 1 out]
    n638 = case shown="No Error" w1029 {
      selector: w1029 -> [_ w1123]
      tunnel: w1026 -> [w1056 _]
      tunnel: w1033 -> [w1051 _]
      tunnel: w1027 -> [w1037 _]
      tunnel: w1025 -> [w1036 _]
      frame No Error {
        # "Receive data"
        n639 = TCP Read(connection ID=w1056, bytes to read=1024, 7:T38."CRLF" ("mode (standard)"), 9:500 ("timeout ms (25000)")) -> (connection ID out=w1048:refnum<k5>, data out=w1053:string, error out=w1050:errorcluster)  [unwired: 1 in]
        n640 = call <vilib>:"Trim Whitespace.vi"("string"=w1053) -> ("trimmed string"=w1052:string)  [unwired: 1 in]
        n641 = case shown="\"abort\"" w1052 {
          selector: w1052 -> [w1086 _ _ _ _]
          tunnel: w1051 -> [w1085 _ _ _ _]
          tunnel: w1050 -> [w1080 _ _ _ _]
          tunnel: [_ "done\r\n" ("data in") w1115 "hello\r\n" ("data in") _] -> w1040
          tunnel: w1037 -> [w1082 w1114 _ _ w1121]
          tunnel: w1036 -> [w1081 w1113 _ _ _]
          tunnel: [w1077 w1111 _ _ _] -> w1038
          frame Default {
            # "check it's an HDF"
            n642 = Get Date/Time In Seconds() -> (seconds since 1Jan1904=w1084:timestamp)
            n643 = String To Path(string=w1086) -> (path=w1078:path)
            n644 = Format Into String(format string="Received \"%s\" from %s at %T", w1086, w1085, w1084) -> (resulting string=w1083:string)  [unwired: 2 in, 1 out]
            n645 = call <vilib>:"H5F_is_hdf.vi"("error in (no error)"=w1080, "path"=w1078) -> ("valid"=w1079:bool)  [unwired: 1 in, 2 out]
            n646 = call <userlib>:"BasicLogger.vi"("text"=w1083) -> ()  [unwired: 6 in, 2 out]
            n647 = case shown="True" w1079 {
              tunnel: w1078 -> [w1090 w1103]
              tunnel: w1082 -> [_ w1105]
              tunnel: [w1092 w1095] -> w1077
              tunnel: w1081 -> [_ w1104]
              frame False {
                n648 = Format Into String(format string="Received file \"%s\" not a valid HDF ", w1090) -> (resulting string=w1089:string)  [unwired: 2 in, 1 out]
                n649 = call <vilib>:"Error Cluster From Error Code.vi"("error message (\"\")"=w1089, "error code (0)"=6042 ("t")) -> ("error out"=w1092:errorcluster)  [unwired: 7 in]
              }
              frame True {
                n650 = call-dynamic "CameraAbort.vi"("CameraBase in"=w1104) -> ("error out"=w1094:errorcluster)  [unwired: 9 in, 1 out]
                n651 = call <vilib>:"Clear Errors.vi"("error in (no error)"=w1094) -> ("error out"=w1093:errorcluster)  [unwired: 6 in]
                n652 = Flush Queue(queue=w1105, error in (no error)=w1093) -> (queue out=w1101:refnum<queue>, error out=w1102:errorcluster)  [unwired: 1 out]
                n653 = flat-sequence {
                  tunnel: w1103 -> [w1106]
                  tunnel: w1102 -> [w1107]
                  tunnel: [w1107] -> w1097
                  frame #0 {
                    n654 = Strip Path(path=w1106) -> (stripped path=w1109:path, name=w1108:string)
                    n655 = local write "working dir"(w1109) -> ()
                    n656 = local write "current file"(w1108) -> ()
                  }
                }
                n657 = Enqueue Element(queue=w1101, element=Imaging_State."Read File", error in (no error)=w1097) -> (queue out=w1099:refnum<queue>, error out=w1096:errorcluster)  [unwired: 1 in, 1 out]
                n658 = Enqueue Element(queue=w1099, element=Imaging_State."Acquire", error in (no error)=w1096) -> (error out=w1095:errorcluster)  [unwired: 1 in, 2 out]
              }
            }
          }
          frame "abort" {
            # "BLACS signals abort"
            # "Kill the queue"
            # "Abort the camera"
            n659 = call-dynamic "CameraAbort.vi"("CameraBase in"=w1113) -> ("error out"=w1111:errorcluster)  [unwired: 9 in, 1 out]
            n660 = call <vilib>:"Clear Errors.vi"("error in (no error)"=w1111) -> ("error out"=w1112:errorcluster)  [unwired: 6 in]
            n661 = Flush Queue(queue=w1114, error in (no error)=w1112) -> ()  [unwired: 3 out]
          }
          frame "state" {
            n662 = local read "state"() -> (w1117:T11)
            n663 = Format Into String(format string="%s\\r\\n", w1117) -> (resulting string=w1115:string)  [unwired: 2 in, 1 out]
          }
          frame "hello" {
            n664 = call <userlib>:"BasicLogger.vi"("text"="Received TCP ping") -> ()  [unwired: 6 in, 2 out]
          }
          frame "done" {
            n665 = Enqueue Element(queue=w1121, element=Imaging_State."Save File") -> ()  [unwired: 2 in, 3 out]
            n666 = call <userlib>:"BasicLogger.vi"("text"="Received \"done\" command") -> ()  [unwired: 6 in, 2 out]
          }
        }
        n667 = case shown="Default" w1040 {
          selector: w1040 -> [w1067 _]
          tunnel: w1048 -> [w1068 w1074]
          tunnel: [w1068 w1071] -> w1044
          tunnel: [w1067 "done\r\n"] -> w1043
          tunnel: [_ w1070] -> w1039
          tunnel: w1038 -> [_ w1069]
          frame Default {
          }
          frame "" {
            # "Make sure it worked"
            # "Send acknowledge response"
            n668 = TCP Write(connection ID=w1074, data in="ok\r\n", 9:500 ("timeout ms (25000)")) -> (connection ID out=w1071:refnum<k5>, error out=w1076:errorcluster)  [unwired: 1 in, 1 out]
            n669 = call <vilib>:"Clear Errors.vi"("error in (no error)"=w1076) -> ()  [unwired: 6 in, 1 out]
            n670 = call <userlib>:"Get_Notifier.vi"("error in"=w1069) -> ("error out"=w1070:errorcluster)  [unwired: 2 in]
          }
        }
        n671 = case shown="No Error" w1039 {
          selector: w1039 -> [w1062 _]
          tunnel: [w1060 w1066] -> w1047
          tunnel: w1043 -> [_ w1066]
          tunnel: w1037 -> [w1058 _]
          tunnel: [w1057 _] -> _
          tunnel: w1036 -> [_ _]
          tunnel: [_ TRUE] -> w1035
          frame Error {
            w1061 = T16 0 items=["no dialog", "OK message", "continue or stop message", "OK message + warnings", "continue/stop + warnings"] ("type of dialog (OK msg:1)")
            # "Kill an acquisition if running (?)"
            # "kill any commands in the queue"
            # "Check if any errors occurred\nIf they did, BLACS will want to know"
            n672 = Flush Queue(queue=w1058) -> ()  [unwired: 1 in, 3 out]
            n673 = call <vilib>:"Clear Errors.vi"() -> ()  [unwired: 7 in, 1 out]
            n674 = call <vilib>:"Simple Error Handler.vi"("type of dialog (OK msg:1)"=w1061, "error in (no error)"=w1062) -> ("error out"=w1059:errorcluster, "message"=w1063:string)  [unwired: 3 in, 3 out]
            n675 = Concatenate Strings("ERROR: " ("string"), w1063) -> (w1060:string)
            n676 = call <userlib>:"BasicErrorLogger.vi"("error in"=w1059) -> ("error out"=w1057:errorcluster)  [unwired: 1 in, 1 out]
          }
          frame No Error {
          }
        }
        n677 = TCP Write(connection ID=w1044, data in=w1047, 9:500 ("timeout ms (25000)")) -> (connection ID out=w1042:refnum<k5>, error out=w1045:errorcluster)  [unwired: 1 in, 1 out]
        n678 = local write "remote"(w1035) -> ()
        n679 = TCP Close Connection(connection ID=w1042, error in (no error)=w1045) -> (error out=w1049:errorcluster)  [unwired: 1 in, 1 out]
        n680 = call <vilib>:"Clear Errors.vi"("error in (no error)"=w1049) -> ()  [unwired: 6 in, 1 out]
      }
      frame Error {
        n681 = call <userlib>:"BasicErrorLogger.vi"("error in"=w1123) -> ()  [unwired: 1 in, 2 out]
      }
    }
  }
  n682 = Stop(stop? (T)=w56) -> ()
  "acquiring" <- w25
